vi "MoD Main-Optimize - HPLC ketene2.vi"() -> ()   [LabVIEW 2015]
uses:
  <vilib>/silver_ctls/ArrayMatrixCluster/Real Matrix NI_Silver.ctl
  <vilib>/ni845x/ni845x.llb/ni845xControl.ctl
  <vilib>/MakerHub/LINX/Public/Peripherals/Analog/Analog Read 1 Chan.vi
  <vilib>/MakerHub/LINX/Public/Peripherals/Analog/Analog Read N Chans.vi
  <vilib>/MakerHub/LINX/Public/Peripherals/Digital/Digital Write 1 Chan.vi
  <vilib>/MakerHub/LINX/Private/Local IO/LinxAnalogRead.vi
  <vilib>/MakerHub/LINX/Public/Utilities/Check Channel.vi
  <vilib>/MakerHub/LINX/Public/Peripherals/Digital/Digital Write N Chans.vi
  <vilib>/MakerHub/LINX/Private/Local IO/LinxDigitalWrite.vi
  <vilib>/addons/control/pid/pid.llb/PID Control Input Filter (DBL).vi
  <vilib>/MakerHub/LINX/Private/Utilties/Generate Error.vi
  <vilib>/addons/control/pid/autopid.llb/PID Online Autotuning (Relay Feedback).vi
  <vilib>/Analysis/Matrix/Numeric/Conversions/Array To Matrix - RA2.vi
  <vilib>/ni845x/ni845x.llb/NI-845x Close Device Reference.vi
  <vilib>/addons/control/pid/NI_PID_autopid.lvlib
  <vilib>/addons/control/pid/NI_PID_pid.lvlib
  <vilib>/Analysis/Matrix/NI_Matrix.lvlib
  <vilib>/MakerHub/LINX/LMH-LINX.lvlib
  <instrlib>/Harvard Apparatus PHD Ultra Series/Harvard Apparatus PHD Ultra Series.lvlib
panel:
  out "Temp SS? 6":bool=TRUE
  out "running?":bool=TRUE
  out "new_reactor_volume":bool[](array[boolean])
  out "new_reactor_length":bool[](array[boolean])
  out "Phase_Sensor_voltage":dbl
  out "P_tot":dbl
  out "pause for ms":bool=TRUE
  out "stop_xl_write":bool=TRUE
  out "Num_exp_till_pause":i32
  out "Syringe_pump?":bool=TRUE
  out "System Error":bool=TRUE
  out "error out":errorcluster
  out "Pump setpoint(ul/min) 6":dbl format="%#_13g"
  out "Pump setpoint(ul/min) 5":dbl format="%#_13g"
  out "Pump setpoint(ul/min) 4":dbl format="%#_13g"
  out "Pump setpoint(ul/min) 3":dbl format="%#_13g"
  out "Pump setpoint(ul/min) 2":dbl format="%#_13g"
  out "Pump setpoint(ul/min) 1":dbl format="%#_13g"
  out "Volume (ul) 5":dbl format="%#_13g"
  out "Volume (ul) 4":dbl format="%#_13g"
  out "Volume (ul) 3":dbl format="%#_13g"
  out "Volume (ul) 2":dbl format="%#_13g"
  out "Volume (ul) 1":dbl format="%#_13g"
  in  "tau 5":dbl format="%#_13g"
  out "tau 4":dbl format="%#_13g"
  out "tau 3":dbl format="%#_13g"
  out "tau 2":dbl format="%#_13g"
  out "tau 1":dbl format="%#_13g"
  out "Reactor Length":dbl format="%#_13g"
  out "Flowrate Sensor 2":dbl format="%#_13g"
  out "Flowrate Sensor 1":dbl format="%#_13g"
  out "Pressure 2":dbl format="%#_13g"
  out "Pressure 1":dbl format="%#_13g"
  out "Temperature Control 5":bool=TRUE
  out "Temperature Control 4":bool=TRUE
  out "Temperature Control 3":bool=TRUE
  out "Temperature Control 2":bool=TRUE
  out "Temperature Control 1":bool=TRUE
  out "Temperature SP 5":dbl format="%#_g'C"
  out "Temperature SP 4":dbl format="%#_g'C"
  out "Temperature SP 3":dbl format="%#_g'C"
  out "Temperature SP 2":dbl format="%#_g'C"
  out "Temperature SP 1":dbl format="%#_g'C"
  in  "Bay Temperature 5":dbl
  in  "SSR Duration 5":dbl
  in  "SSR Duration 4":dbl
  in  "SSR Duration 3":dbl
  in  "SSR Duration 2":dbl
  in  "SSR Duration 1":dbl
  in  "Total Product Amount":dbl=1.0 format="%#_gml"
  out "Setup Error":bool=TRUE
  out "Error Message":string
  out "ID CTR":i32
  in  "Tab Control":T1(tab)
  out "Reagent pic 5":picture
  in  "reagent name 5":string="HCl"
  out "Reagent Pic 4":picture
  in  "reagent name 4":string="ethylaluminum dichloride"
  out "Reagent Pic 3":picture
  in  "reagent  name 3":string="cyclohexene"
  in  "Product name":string="55662-89-0"
  in  "reagent name 1":string="Acyl Chloride "
  out "Reagent Pic 1":picture
  in  "Vr5":dbl format="%#_guL"
  in  "Vr4":dbl=400.0 format="%#_guL"
  in  "Vr3":dbl=800.0 format="%#_guL"
  in  "Vr2":dbl format="%#_guL"
  in  "Vr1":dbl format="%#_guL"
  in  "System decide help Button":bool
  in  "Reaction Scheme Confirm":bool
  in  "Synthesis Route Array":string[][](array[string])=[["Acyl Chloride + INTSD", ".5", "PhB(OH)2", "", "", ""], ["Tributyl amine", "4.2", "-", "-", "-", "-"], ["ethylaluminum dichloride", "1", "-", "-", "-", "-"], ["HCl", "", "-", "-", "-", "-"], ["", "", "-", "-", "-", "-"], ["", "", "-", "-", "-", "-"]]
  in  "System decide help Button 2":bool
  out "Setup Confirm":bool=TRUE
  in  "BAY 1":u16(ring) items=["               Bypass", "         Heated Reactor", "    Small Heated Reator", "         Cooled Reactor", "      Packed Bed Reactor", "          Photo Reactor", "             Separator"]
  in  "BAY 5":u16(ring)=6 items=["               Bypass", "         Heated Reactor", "    Small Heated Reactor", "         Cooled Reactor", "     Packed Bed Reactor", "         Photo Reactor", "             Separator"]
  in  "BAY 4":u16(ring)=1 items=["                Bypass", "         Heated Reactor", "    Small Heated Reactor", "         Cooled Reactor", "     Packed Bed Reactor", "         Photo Reactor", "             Separator"]
  in  "BAY 3":u16(ring)=2 items=["               Bypass", "         Heated Reactor", "    Small Heated Reactor", "         Cooled Reactor", "     Packed Bed Reactor", "          Photo Reactor", "             Separator"]
  in  "BAY 2":u16(ring)=2 items=["               Bypass", "         Heated Reactor", "    Small Heated Reactor", "         Cooled Reactor", "      Packed Bed Reactor", "          Photo Reactor", "             Separator"]
  out "Reagent Pic 2":picture
  out "Product Pic":picture
  in  "reagent name 2":string="Tributyl amine"
  in  "reagent name 6":string
  out "Reagent Pic 6":picture
  in  "System Parameters Help Button":bool
  out "Setup Confirm 2":bool
  in  "System Parameters Confirm Button":bool
  in  "Bay Parameters":T2={"Bay 1 "={"Pump 1 Flowrate"=0.0, "optimize_temp"=FALSE, "optimize_tau"=TRUE, "Run at set flowrate"=FALSE, "Pump 2 Flowrate"=0.0, "Temperature Params"=[40.0, 100.0, 100.0], "pump params 1"=[46.3, 463.0, 325.0], "pump params 2"=[11.5, 115.0, 325.0], "Temperature"=0.0, "Run at set temperature"=FALSE}, "Bay 2 "={"Pump 3 Flowrate"=0.0, "optimize_temp"=FALSE, "optimize_tau"=TRUE, "Run at set flowrate"=FALSE, "Temperature Params"=[40.0, 100.0, 100.0], "Resisdence time params"=[4.69, 46.9, 650.0], "pump_at_ratio"=FALSE, "pump_num_ratio"=4.0, "Temperature"=0.0, "Run at set temperature"=FALSE}, "Bay 3 "={"Pump 4 Flowrate"=100.0, "optimize_temp"=TRUE, "optimize_tau"=TRUE, "Run at set flowrate"=FALSE, "Temperature Params"=[30.0, 120.0, 100.0], "Resisdence time params"=[23.15, 231.5, 0.0], "pump_at_ratio"=FALSE, "pump_num_ratio"=1.0, "Temperature "=0.0, "Run at set temperature"=FALSE}, "Bay 4 "={"Pump 5 Flowrate"=40.0, "Run at set flowrate"=FALSE, "optimize_temp"=FALSE, "optimize_tau"=FALSE, "Resisdence time params"=[40.6, 406.0, 225.0], "Temperature Params"=[40.0, 100.0, 80.0], "pump_at_ratio"=FALSE, "pump_num_ratio"=2.0, "Temperature"=0.0, "Run at set temperature"=FALSE}, "Bay 5 "={"Pump 6 Flowrate"=0.0, "Run at set flowrate"=FALSE, "optimize_temp"=FALSE, "optimize_tau"=FALSE, "Resisdence time params"=[7.62, 114.27, 0.0], "Temperature Params"=[0.0, 0.0, 0.0], "pump_at_ratio"=TRUE, "pump_num_ratio"=2.0, "Temperature"=0.0, "Run at set temperature"=FALSE}, "Excel File Name"="C:\\Users\\HPLC\\Dropbox (MIT)\\MoD Files\\Data\\Ketene04222018", "hplc File Name"="C:\\Chem32\\1\\Data\\MOD", "Matlab File"="C:\\Users\\HPLC\\Dropbox (MIT)\\MoD Files\\Data\\Ketene04222018_1", "Syringe for Pump 2?"=TRUE, "Num_conditons_per_wait"=2.0, "Continue from previous optimization?"=FALSE, "Total Number of Experiments 2"=45.0, "Hplc Wait time(min)"=14.0, "increas_decrease_hplc_peak"=FALSE, "Internal Standard?"=TRUE, "ISTD start"=5.0, "ISTD end"=6.0, "hplc_start"=13.0, "hplc_end"=13.45, "throughput_yield"=TRUE} {"Hplc Wait time(min)" format="%#_13g"; "Bay 5"."Temperature Params" format="%#_g'C"; "Bay 4"."Temperature Params" format="%#_g'C"; "Bay 3"."Temperature Params" format="%#_g'C"; "Bay 2"."Temperature Params" format="%#_g'C"; "Bay 1"."Temperature Params" format="%#_g'C"}
  out "System Confirm Not Clicked":string
  out "best_exp_num":dbl=1.0
  out "temperature_best":dbl[](array[numeric])
  out "Flowrates(ul/min)_best":dbl[](array[numeric])
  out "System Status":u16(ring)=2 caption="Sy" items=["System  Error", "System Running", "System Standby"]
  out "Current Experiment":dbl=1.0
  out "Total Number of Experiments":dbl=33.0
  out "Phase Sensor Chart":T3(graph)
  out "HPLC Analysis":bool
  out "Equlibrating Temperature":bool
  out "Flushing System":bool
  out "Calculate condition":bool
  out "Temperature 5":dbl format="%#_g'C"
  out "Temperature 4":dbl format="%#_g'C"
  out "Temperature 3":dbl format="%#_g'C"
  out "Temperature 2":dbl format="%#_g'C"
  out "Temperature 1":dbl format="%#_g'C"
  out "Flowrate Chart":T4(graph)
  out "Teperature Chart":T3(graph)
  out "Pump Setpoints Chart":T3(graph)
  out "Pressure Chart":T3(graph)
  out "Optimization_loop_index":i32
  out "curr_wait_time":dbl
  out "total_flush_time":dbl
  out "Temp SS? 5":bool=TRUE
  out "Temp SS? 4":bool=TRUE
  out "Temp SS? 3":bool=TRUE
  out "Temp SS? 2":bool=TRUE
  out "Temp SS? 1":bool=TRUE
  out "System Flushed?":bool
  out "stop_button clicked":bool
  in  "Pump Addresses":string[](array[string])=["g", "e", "j", "i", "f", "h"]
  out "experiment history":T5
  in  "Number of System Flushes per condtion":dbl=2.5
  in  "calculate volume 3":bool=TRUE
  in  "calculate volume 2":bool=TRUE
  in  "calculate volume 1":bool=TRUE
  in  "calculate volume 4":bool=TRUE
  in  "calculate volume 5":bool
  in  "Extra system dead volume":dbl format="%#_gul"
  in  "new reactor length? 1":bool
  in  "tube_length(in)":dbl[](array[numeric])=[188.0, 188.0, 10.0, 10.0, 10.0]
  out "Pause Before Analysis":bool
  out "Chiller COMM Port":bool
  out "Arduino COMM Port 2":bool
  out "Temperature Sensor COMM Port":bool
  out "Flow Rate":bool
  out "Pressure":bool
  out "Pump COMM Port":bool
  in  "COMM Port :: Milligat Pumps":refnum<visa-resource-name>="COM10"
  in  "Arduino COMM Port":refnum<visa-resource-name>="COM3"
  in  "Sample Valve COMM::Port":refnum<visa-resource-name>="COM4"
  in  "COMM Port:: Harvard Syringe Pump":refnum<visa-resource-name>="COM5"
  in  "tube_id(in)":enum16{".01", ".02", ".03", ".04"}[](array[ring])=[enum.".03", enum.".03", enum.".03", enum.".03", enum.".03"]
  out "Total System Resisdence Time(min)":dbl
  in  "Debug_run_button":bool
  in  "new reactor length? 2":bool
  in  "new reactor length? 3":bool
  in  "new reactor length? 4":bool
  in  "new reactor length? 5":bool
  in  "IR Sensor Device":T6="USB0::0x3923::0x7514::01B3FF21::RAW"
  out "Stop":bool=TRUE
  in  "Run_Stop_cluster":T7
  # "Molecules on Demand"
  # "Synthetic Route"
  # "5"
  # "6"
  # "4"
  # "Product"
  # "1"
  # "2"
  # "3"
  # "Reagent List"
  # "Concentration(M)"
  # "Molecule"
  # "1"
  # "1"
  # "2"
  # "2"
  # "3"
  # "3"
  # "4"
  # "4"
  # "5"
  # "6"
  # "5"
  # "6"
  # "Product"
  # "Reactor Volume:"
  # "Optimization Parameters"
  # "Pause after"
  # "Experiments"
  # "Optimize for"
  # "to"
  # "of HPLC Peak from"
  # "from"
  # "to"
  # "min"
  # "min"
  # "HPLC runtime"
  # "# Iterations"
  # "Reporting"
  # "Excel Output File Name"
  # "HPLC File Path"
  # "MATLAB File Path"
  # "Temperature"
  # "Flowrate(ul/min)"
  # "Lower Bound"
  # "Upper Bound"
  # "Optimize?"
  # "-or-"
  # "Run at"
  # "times incoming flow"
  # "Setpoint"
  # "Temperature"
  # "Flowrate(ul/min)"
  # "Lower Bound"
  # "Upper Bound"
  # "Optimize?"
  # "-or-"
  # "Run at"
  # "times incoming flow"
  # "Setpoint"
  # "Temperature"
  # "Flowrate(ul/min)"
  # "Lower Bound"
  # "Upper Bound"
  # "Optimize?"
  # "-or-"
  # "Run at"
  # "times incoming flow"
  # "Setpoint"
  # "Temperature"
  # "Flowrate 3 (ul/min)"
  # "Lower Bound"
  # "Upper Bound"
  # "Optimize?"
  # "-or-"
  # "Run at"
  # "times incoming flow"
  # "Setpoint"
  # "Temperature"
  # "Flowrate 1(ul/min)"
  # "Flowrate 2(ul/min)"
  # "Lower Bound"
  # "Upper Bound"
  # "Optimize?"
  # "Setpoint"
  # "Pressure (psi)"
  # "System Status"
  # "Temperature('C)"
  # "BAY"
  # "1"
  # "2"
  # "3"
  # "4"
  # "5"
  # "Pump Flowrate Setpoint(ul/min)"
  # "Flowrate (ul/min)"
  # "Phase Sensor"
  # "Current Experiment"
  # "Temperature('C)"
  # "Flowrate(ul/min)"
  # "Exp"
  # "Current Best Condition"
  # "Time to reach steady state:"
  # "Current Wait Time:"
  # "Experimental Steps"
  # "Calculated New Conditions"
  # "Steady State"
  # "Analyzed HPLC"
  # "Equilibrated Temperature"
  # "Tube Length (cm)"
  # "Bay"
  # "Tube ID (in)"
  # "Calculate Volume"
  # "Use new tube length"
  # "1."
  # "2."
  # "3."
  # "4."
  # "5."
  # "Reactor Lengths\n*Heated Reactor - 188cm * Small Reactor - 99cm * Bypass - 10cm * Separator - *"
  # "1"
  # "2"
  # "3"
  # "4"
  # "5"
  # "All Experimental Data"
  # "6"
  # "P1"
  # "P2"
  # "P3"
  # "P4"
  # "P5"
  # "P6"
  # "T1"
  # "T2"
  # "T3"
  # "T4"
  # "T5"
  # "Obj_fun"
  # "HPLC_Data"
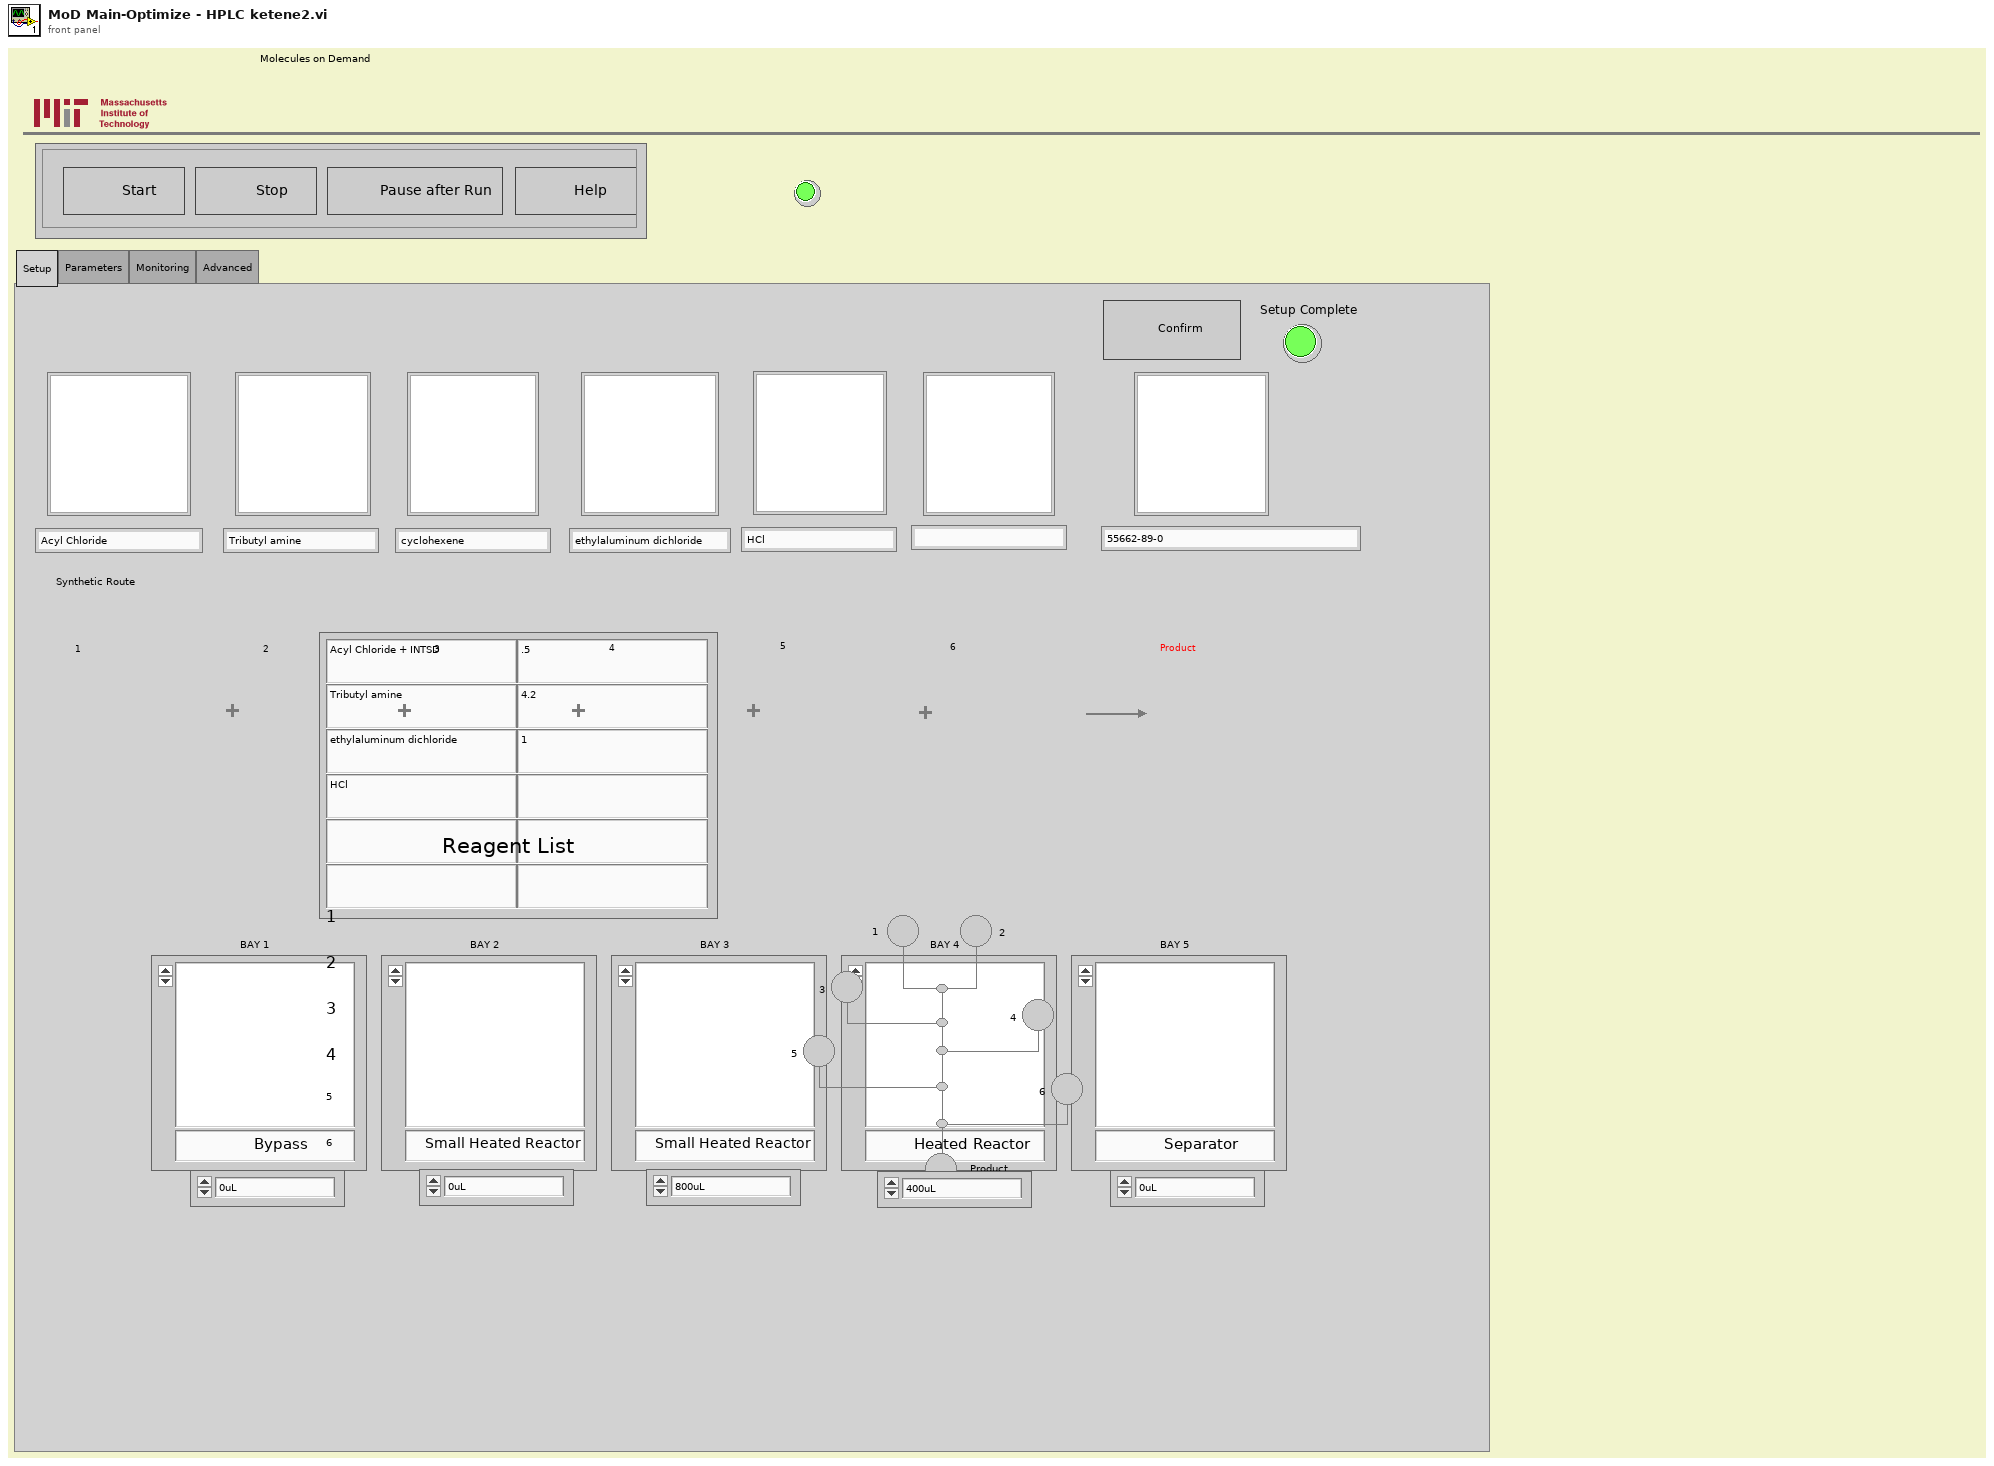
[diagram p1: front panel]
types:
  T1 = enum32{"Setup", "Parameters", "Monitoring", "Advanced"}
  T2 = cluster{"Bay 1 ":cluster{"Pump 1 Flowrate":dbl, "optimize_temp":bool, "optimize_tau":bool, "Run at set flowrate":bool, "Pump 2 Flowrate":dbl, "Temperature Params":dbl[], "pump params 1":dbl[], "pump params 2":dbl[], "Temperature":dbl, "Run at set temperature":bool}, "Bay 2 ":cluster{"Pump 3 Flowrate":dbl, "optimize_temp":bool, "optimize_tau":bool, "Run at set flowrate":bool, "Temperature Params":dbl[], "Resisdence time params":dbl[], "pump_at_ratio":bool, "pump_num_ratio":dbl, "Temperature":dbl, "Run at set temperature":bool}, "Bay 3 ":cluster{"Pump 4 Flowrate":dbl, "optimize_temp":bool, "optimize_tau":bool, "Run at set flowrate":bool, "Temperature Params":dbl[], "Resisdence time params":dbl[], "pump_at_ratio":bool, "pump_num_ratio":dbl, "Temperature ":dbl, "Run at set temperature":bool}, "Bay 4 ":cluster{"Pump 5 Flowrate":dbl, "Run at set flowrate":bool, "optimize_temp":bool, "optimize_tau":bool, "Resisdence time params":dbl[], "Temperature Params":dbl[], "pump_at_ratio":bool, "pump_num_ratio":dbl, "Temperature":dbl, "Run at set temperature":bool}, "Bay 5 ":cluster{"Pump 6 Flowrate":dbl, "Run at set flowrate":bool, "optimize_temp":bool, "optimize_tau":bool, "Resisdence time params":dbl[], "Temperature Params":dbl[], "pump_at_ratio":bool, "pump_num_ratio":dbl, "Temperature":dbl, "Run at set temperature":bool}, "Excel File Name":string, "hplc File Name":string, "Matlab File":string, "Syringe for Pump 2?":bool, "Num_conditons_per_wait":dbl, "Continue from previous optimization?":bool, "Total Number of Experiments 2":dbl, "Hplc Wait time(min)":dbl, "increas_decrease_hplc_peak":bool, "Internal Standard?":bool, "ISTD start":dbl, "ISTD end":dbl, "hplc_start":dbl, "hplc_end":dbl, "throughput_yield":bool}
  T3 = cluster{"[0]":dbl, "[1]":dbl, "[2]":dbl, "[3]":dbl, "[4]":dbl, "[5]":dbl, "[6]":dbl, "[7]":dbl, "[8]":dbl}
  T4 = cluster{"[0]":i32, "[1]":i32, "[2]":i32, "[3]":i32, "[4]":i32, "[5]":i32, "[6]":i32, "[7]":i32, "[8]":i32}
  T5 = typedef "Real Matrix NI_Silver.ctl" = dbl[][]
  T6 = typedef "ni845xControl.ctl" = refnum<k21>
  T7 = cluster{"Stop":bool, "Run":bool, "Stop Run Button":bool, "Help Button":bool}
  T8 = cluster{"Proportional gain Kc":dbl, "Integral time Ti (sec)":dbl, "Derivative time Ti (sec)":dbl}
  T9 = cluster{"type of controller":enum16{"P", "PI", "PID"}, "relay cycles":i32, "relay amplitude":dbl, "control specifications":enum16{"Fast", "Normal", "Slow"}, "PV noise level":dbl}
  T10 = typedef "LMH-LINX.lvlib/LINX Ref.ctl" = cluster{"IO":T11, "Interface":T12, "LINX Device Config":T13}
  T11 = typedef "LMH-LINX.lvlib/Platform.ctl" = enum16{"Remote", "Local"}
  T12 = typedef "LMH-LINX.lvlib/Interface.ctl" = enum16{"Serial", "TCP"}
  T13 = typedef "LMH-LINX.lvlib/Device.lvlib/LINX Device Config.ctl" = cluster{"Interface":T12, "COM Port":refnum<visa-resource-name>, "TCP Configuration":T14, "Device Family":u8, "Device ID":u8, "Device Name":string, "TCP Ref":refnum<k5>, "Channels":T15}
  T14 = typedef "LMH-LINX.lvlib/Device.lvlib/TCP Config.ctl" = cluster{"IP Address":string, "Port":u16}
  T15 = typedef "LMH-LINX.lvlib/Channels.ctl" = cluster{"DI":u8[], "DO":u8[], "AI":u8[], "AO":u8[], "PWM":u8[], "QE":u8[], "UART":u8[], "I2C 2":u8[], "SPI":u8[], "CAN":u8[], "Servo":u8[], "AI Ref (V)":dbl, "AI Resolution (Bits)":u8, "AO Ref (V)":dbl, "AO Resolution (Bits)":u8}
  T16 = typedef "imagedata.ctl" = cluster{"image type":i32, "image depth":i32, "image":u8[], "mask":u8[], "colors":u32[], "Rectangle":cluster{"left":i16, "top":i16, "right":i16, "bottom":i16}}
  T17 = cluster{"proportional gain (Kc)":dbl, "integral time (Ti, min)":dbl, "derivative time (Td, min)":dbl}
  T18 = typedef "NI_Matrix.lvlib/RealMatrix.ctl" = dbl[][]
  T19 = enum16{"Left Button", "Center Button", "Right Button", "Window Close"}
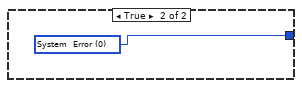
[diagram p4: hidden frame]
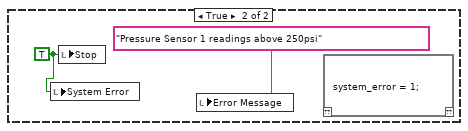
[diagram p6: hidden frame]
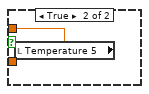
[diagram p7: hidden frame]
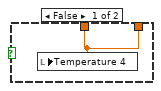
[diagram p8: hidden frame]
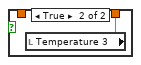
[diagram p9: hidden frame]
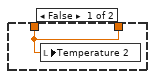
[diagram p10: hidden frame]
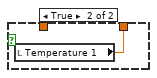
[diagram p11: hidden frame]
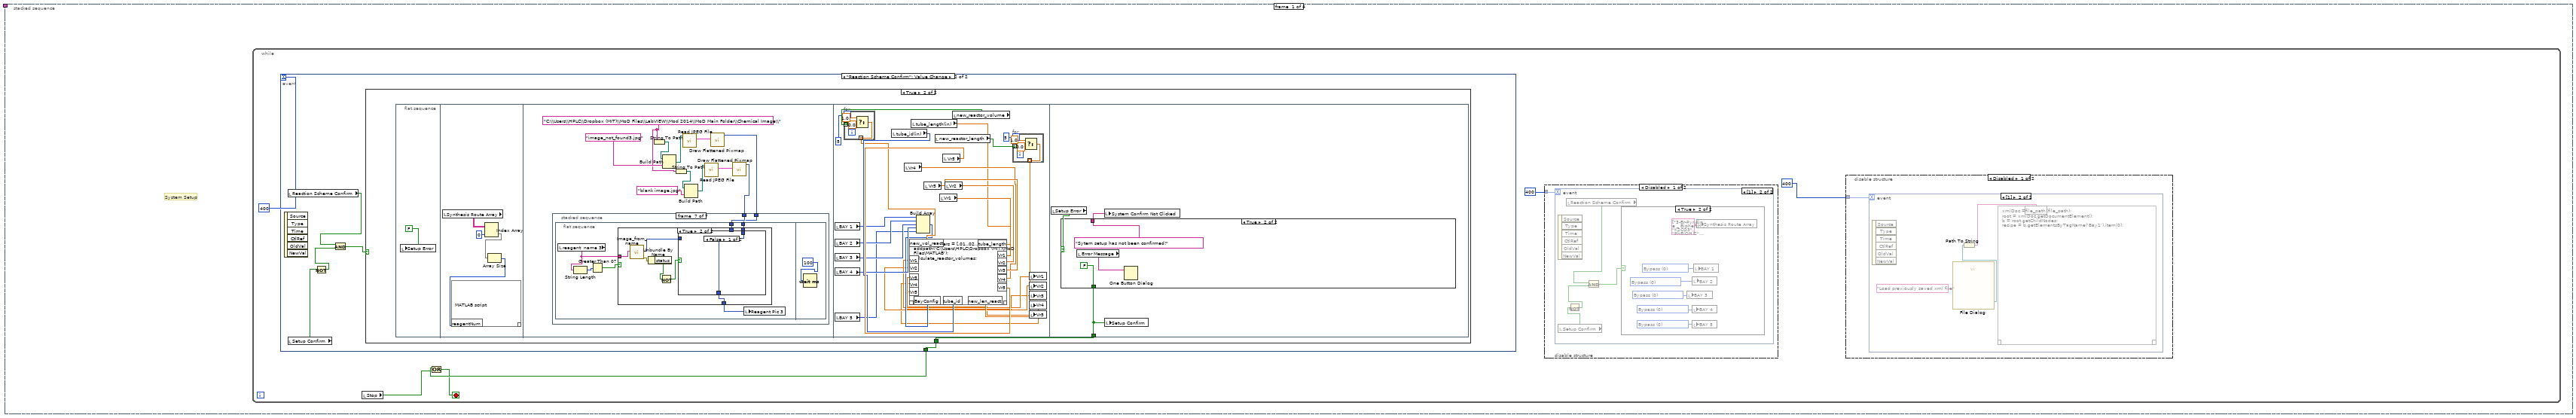
[diagram p12: hidden frame]
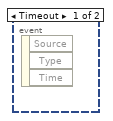
[diagram p13: hidden frame]
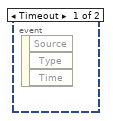
[diagram p15: hidden frame]
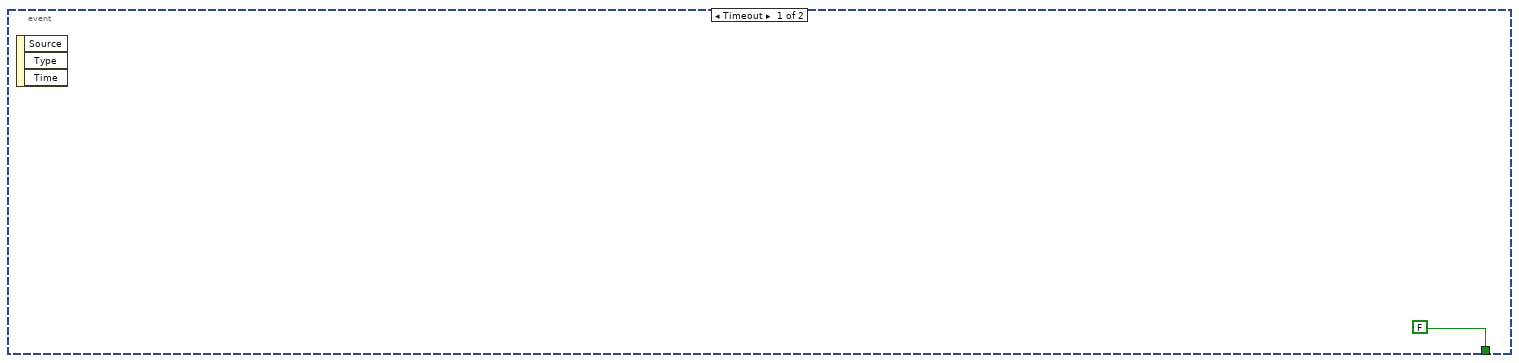
[diagram p18: hidden frame]
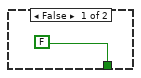
[diagram p19: hidden frame]
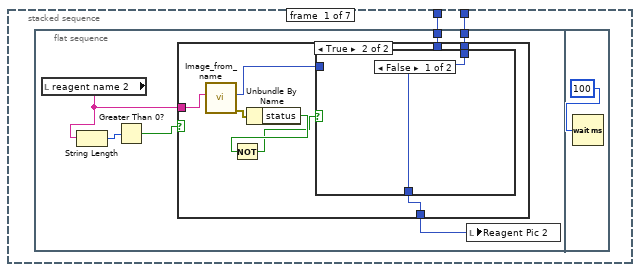
[diagram p20: hidden frame]
diagram:
  # "Assume User always uses the first bay first"
  n1 = flat-sequence {
    tunnel: ["COMM Port :: Milligat Pumps"] -> w9
    tunnel: ["Arduino COMM Port"] -> w8
    tunnel: [w11] -> w5
    tunnel: ["Bay Parameters"] -> w4
    tunnel: [w60] -> w10
    tunnel: w9 -> [w60]
    tunnel: w8 -> [w48]
    tunnel: [w54] -> w7
    tunnel: [w52] -> w6
    tunnel: w5 -> [w52]
    tunnel: w4 -> [w50]
    tunnel: [w47] -> w3
    tunnel: w10 -> [w66]
    tunnel: w7 -> [w65]
    tunnel: w6 -> [w63]
    tunnel: w3 -> [w61]
    tunnel: [w61] -> w1
    tunnel: [w1409] -> w2
    tunnel: w1 -> [w1409]
    tunnel: w2 -> [w1410]
    frame #0 {
      w36 = FALSE ("Equlibrating Temperature")
      n2 = script code="TempArr1=[23 23 23 23 23 23 23 23 23 23]';\nTempArr2=[23 23 23 23 23 23 23 23 23 23]';\nTempArr3=[23 23 23 23 23 23 23 23 23 23]';\nTempArr4=[23 23 23 23 23 23 23 23 23 23]';\nTempArr5=[23 23 23 23 23 23 23 23 23 23]';\nTempArrLED=[23 23 23 23 23 23 23 23 23 23]';\ntemp_error1 =0;\ntemp_error2 =0;\ntemp_error3 =0;\ntemp_error4 =0;\ntemp_error5 =0;\ntemp_check1 = 0;\ntemp_check2 = 0;\ntemp_check3 = 0;\ntemp_check4 = 0;\ntemp_check5 = 0;\nT1=23;\nT2=23;\nT3=23;\nT4=23;\nT5=23;"() -> ()  [unwired: 1 in, 1 out]
      n3 = Build Array("calculate volume 1", "calculate volume 2", "calculate volume 3", "calculate volume 4", "calculate volume 5") -> (→"new_reactor_volume":bool[])
      n4 = Build Array("new reactor length? 1", "new reactor length? 2", "new reactor length? 3", "new reactor length? 4", "new reactor length? 5") -> (→"new_reactor_length":bool[])
      n5 = call <vilib>:"Initialize.vi"("VISA resource name"="COMM Port:: Harvard Syringe Pump") -> ("VISA resource name out"=w11:refnum<visa-resource-name>)  [unwired: 9 in, 1 out]
      "Stop" <- FALSE ("Stop")
      "ID CTR" <- 0
      "Setup Confirm" <- FALSE ("Setup Confirm")
      "Error Message" <- "System shutdown sucessfully. No errors to report." ("Error Message")
      "Setup Error" <- FALSE ("Setup Error")
      "Reactor Length" <- 10.5
      "System Error" <- FALSE ("System Error")
      "Num_exp_till_pause" <- 0 ("Num_exp_till_pause")
      "Equlibrating Temperature" <- w36
      "Calculate condition" <- w36
      "Flushing System" <- w36
      "HPLC Analysis" <- w36
      "stop_xl_write" <- FALSE ("stop_xl_write")
      "Pump setpoint(ul/min) 1" <- 0.0 ("Pump setpoint(ul/min) 1")
      "Pump setpoint(ul/min) 2" <- 0.0 ("Pump setpoint(ul/min) 2")
      "Pump setpoint(ul/min) 4" <- 0.0 ("Pump setpoint(ul/min) 4")
      "Pump setpoint(ul/min) 6" <- 0.0 ("Pump setpoint(ul/min) 6")
      "Pump setpoint(ul/min) 3" <- 0.0 ("Pump setpoint(ul/min) 3")
      "Pump setpoint(ul/min) 5" <- 0.0 ("Pump setpoint(ul/min) 5")
      "pause for ms" <- FALSE ("pause for ms")
      "Setup Confirm 2" <- FALSE ("Setup Confirm 2")
      "running?" <- FALSE ("running?")
    }
    frame #1 {
      w49 = FALSE
      w59 = 23
      (unwired) path "C:/Users/User1/Documents/Lab/MoD/Images"
      n6 = disable-structure shown="Disabled" {
        frame Disabled {
          n7 = local read "BAY 2"() -> ()  [unwired: 1 out]
          n8 = local read "BAY 3"() -> ()  [unwired: 1 out]
          n9 = local read "BAY 4"() -> ()  [unwired: 1 out]
          n10 = local read "BAY 5"() -> ()  [unwired: 1 out]
          n11 = local read "BAY 1"() -> ()  [unwired: 1 out]
        }
        frame Enabled {
        }
      }
      n12 = local write "Debug_run_button"(TRUE) -> ()
      n13 = call <vilib>:"Initialize.vi"("Serial Port"=w48) -> ("LINX Resource"=w47:T10)  [unwired: 8 in, 2 out]
      n14 = local write "System Parameters Confirm Button"(w49) -> ()
      n15 = local write "Setup Confirm 2"(w49) -> ()
      n16 = Unbundle By Name(w50) -> ("Syringe for Pump 2?"=→"Syringe_pump?":bool)
      n17 = local write "Temperature 1"(w59) -> ()
      n18 = local write "Temperature 2"(w59) -> ()
      n19 = local write "Temperature 3"(w59) -> ()
      n20 = local write "Temperature 4"(w59) -> ()
      n21 = local write "Temperature 5"(w59) -> ()
      n22 = local write "Temperature SP 1"(w59) -> ()
      n23 = local write "Temperature SP 2"(w59) -> ()
      n24 = local write "Temperature SP 3"(w59) -> ()
      n25 = local write "Temperature SP 4"(w59) -> ()
      n26 = local write "Temperature SP 5"(w59) -> ()
      n27 = Current VI's Path() -> (path=w58:path)
      n28 = Strip Path(path=w58) -> (stripped path=w56:path)  [unwired: 1 out]
      n29 = Strip Path(path=w56) -> (stripped path=w55:path)  [unwired: 1 out]
      n30 = Build Path(base path=w55, name or relative path="MATLAB") -> (appended path=w54:path)
    }
    frame #2 {
      # "Main Help Dialog Popup"
      n31 = while {
        stop <- w1403 stop-if-true
        n32 = event shown="[6] \"Run_Stop_cluster.Run\": Value Change" {
          selector: _ -> [_ _ _ _ _ _ _]
          dyn-events: _ -> [_ _ _ _ _ _ _]
          timeout: 100 -> [_ _ _ _ _ _ _]
          event Timeout {
            n33 = event-data() -> ()  [unwired: 1 in, 3 out]
          }
          event "Run_Stop_cluster.Help Button": Value Change {
            n34 = local read "Run_Stop_cluster"() -> (w1406:T7)
            n35 = event-data() -> ()  [unwired: 1 in, 4 out]
            n36 = Unbundle By Name(w1406) -> ("Help Button"=w1405:bool)
            n37 = case shown="True" w1405 {
              frame False {
              }
              frame True {
                n38 = call "help.vi"() -> ()  [unwired: 11 in]
              }
            }
          }
          event "System decide help Button": Value Change {
            n39 = event-data() -> ()  [unwired: 1 in, 5 out]
            n40 = call "help_synthesis_man-auto_instructions.vi"() -> ()  [unwired: 12 in]
          }
          event "System Parameters Help Button": Value Change {
            n41 = event-data() -> ()  [unwired: 1 in, 5 out]
            n42 = call "help_parameters_setup.vi"() -> ()  [unwired: 12 in]
          }
          event "System decide help Button 2": Value Change {
            n43 = event-data() -> ()  [unwired: 1 in, 5 out]
            n44 = call "help_synthesis_route_instructions.vi"() -> ()  [unwired: 12 in]
          }
          event "Run_Stop_cluster.Stop": Value Change {
            n45 = event-data() -> ()  [unwired: 1 in, 5 out]
            n46 = local write "Stop"(TRUE) -> ()
          }
          event "Run_Stop_cluster.Run": Value Change {
            n47 = event-data() -> ()  [unwired: 1 in, 5 out]
            n48 = local write "running?"(TRUE) -> ()
          }
        }
        n49 = local read "Stop"() -> (w1403:bool)
      }
      n50 = stacked-sequence {
        tunnel: w66 -> [_ _ _ _]
        tunnel: w65 -> [_ w432 _ _]
        tunnel: w63 -> [_ _ _ w599]
        tunnel: w61 -> [_ _ _ w597]
        frame #0 {
          # "System Setup"
          n51 = while {
            stop <- w207 stop-if-true
            n52 = event shown="[1] \"Reaction Scheme Confirm\": Value Change" {
              selector: _ -> [_ _]
              dyn-events: _ -> [_ _]
              timeout: 400 -> [_ _]
              tunnel: [FALSE w227] -> w209
              event Timeout {
                n53 = event-data() -> ()  [unwired: 1 in, 3 out]
              }
              event "Reaction Scheme Confirm": Value Change {
                n54 = event-data() -> ()  [unwired: 1 in, 6 out]
                n55 = local read "Reaction Scheme Confirm"() -> (w231:bool)
                n56 = local read "Setup Confirm"() -> (w229:bool)
                n57 = Not(x=w229) -> (.not. x?=w228:bool)
                n58 = And(x=w231, y=w228) -> (x .and. y?=w230:bool)
                n59 = case shown="True" w230 {
                  tunnel: [FALSE w233] -> w227
                  frame False {
                  }
                  frame True {
                    n60 = flat-sequence {
                      tunnel: [w422] -> w233
                      frame #0 {
                        n61 = local write "Setup Error"(FALSE) -> ()
                      }
                      frame #1 {
                        n62 = local read "Synthesis Route Array"() -> (w237:string[][])
                        n63 = Index Array(array=w237, index (col)=0 ("disabled index (col)")) -> (element=w235:string[])  [unwired: 1 in]
                        n64 = Array Size(array=w235) -> (size(s)=w238:i32)
                        n65 = script code="MATLAB script"("reagentNum"=w238) -> ()  [unwired: 1 in, 1 out]
                      }
                      frame #2 {
                        w241 = "C:\\Users\\HPLC\\Dropbox (MIT)\\MoD Files\\LabVIEW\\Mod 2014\\MoD Main Folder\\Chemical Image\\" ("string")
                        n66 = String To Path(string=w241) -> (path=w247:path)
                        n67 = Build Path(base path=w247, name or relative path="image_not_found3.jpg") -> (appended path=w246:path)
                        n68 = String To Path(string=w241) -> (path=w244:path)
                        n69 = call <vilib>:"Read JPEG File.vi"("path to JPEG file"=w246) -> ("image data"=w249:T16)  [unwired: 1 in, 9 out]
                        n70 = Build Path(base path=w244, name or relative path="blank image.jpg") -> (appended path=w242:path)
                        n71 = call <vilib>:"Read JPEG File.vi"("path to JPEG file"=w242) -> ("image data"=w245:T16)  [unwired: 1 in, 9 out]
                        n72 = call <vilib>:"Draw Flattened Pixmap.vi"("image data"=w249) -> ("new picture"=w240:picture)  [unwired: 3 in, 5 out]
                        n73 = call <vilib>:"Draw Flattened Pixmap.vi"("image data"=w245) -> ("new picture"=w239:picture)  [unwired: 3 in, 5 out]
                        n74 = stacked-sequence {
                          tunnel: w240 -> [w251 w271 w291 w311 w331 w350 w370]
                          tunnel: w239 -> [w250 w270 w290 w310 w330 w351 w371]
                          frame #0 {
                            n75 = flat-sequence {
                              tunnel: w251 -> [w257]
                              tunnel: w250 -> [w255]
                              frame #0 {
                                n76 = local read "reagent name 2"() -> (w253:string)
                                n77 = String Length(string=w253) -> (length=w256:i32)
                                n78 = Greater Than 0?(x=w256) -> (x > 0?=w254:bool)
                                n79 = case shown="True" w254 {
                                tunnel: w257 -> [_ w263]
                                tunnel: w255 -> [w258 _]
                                tunnel: [w258 w262] -> w252
                                tunnel: w253 -> [_ w261]
                                frame False {
                                }
                                frame True {
                                n80 = call "Image_from_name.vi"("Chemical Name"=w261) -> ("error out"=w264:errorcluster, "Downloaded Picture"=w265:picture)  [unwired: 8 in, 1 out]
                                n81 = Unbundle By Name(w264) -> ("status"=w260:bool)
                                n82 = Not(x=w260) -> (.not. x?=w259:bool)
                                n83 = case shown="False" w259 {
                                tunnel: w265 -> [_ w268]
                                tunnel: [w266 w267] -> w262
                                tunnel: w263 -> [w266 _]
                                frame False {
                                }
                                frame True {
                                n84 = call <vilib>:"Draw Flattened Pixmap.vi"("picture"=w268) -> ("new picture"=w267:picture)  [unwired: 8 in]
                                }
                                }
                                }
                                }
                                n85 = local write "Reagent Pic 2"(w252) -> ()
                              }
                              frame #1 {
                                n86 = Wait (ms)(milliseconds to wait=100) -> ()  [unwired: 1 out]
                              }
                            }
                          }
                          frame #1 {
                            n87 = flat-sequence {
                              tunnel: w271 -> [w277]
                              tunnel: w270 -> [w275]
                              frame #0 {
                                n88 = local read "reagent name 1"() -> (w272:string)
                                n89 = String Length(string=w272) -> (length=w276:i32)
                                n90 = Greater Than 0?(x=w276) -> (x > 0?=w274:bool)
                                n91 = case shown="True" w274 {
                                tunnel: w277 -> [_ w283]
                                tunnel: w275 -> [w278 _]
                                tunnel: [w278 w282] -> w273
                                tunnel: w272 -> [_ w281]
                                frame False {
                                }
                                frame True {
                                n92 = call "Image_from_name.vi"("Chemical Name"=w281) -> ("error out"=w284:errorcluster, "Downloaded Picture"=w285:picture)  [unwired: 8 in, 1 out]
                                n93 = Unbundle By Name(w284) -> ("status"=w280:bool)
                                n94 = Not(x=w280) -> (.not. x?=w279:bool)
                                n95 = case shown="True" w279 {
                                tunnel: w285 -> [_ w288]
                                tunnel: [w286 w287] -> w282
                                tunnel: w283 -> [w286 _]
                                frame False {
                                }
                                frame True {
                                n96 = call <vilib>:"Draw Flattened Pixmap.vi"("picture"=w288) -> ("new picture"=w287:picture)  [unwired: 8 in]
                                }
                                }
                                }
                                }
                                n97 = local write "Reagent Pic 1"(w273) -> ()
                              }
                              frame #1 {
                                n98 = Wait (ms)(milliseconds to wait=100) -> ()  [unwired: 1 out]
                              }
                            }
                          }
                          frame #2 {
                            n99 = flat-sequence {
                              tunnel: w291 -> [w297]
                              tunnel: w290 -> [w295]
                              frame #0 {
                                n100 = local read "Product name"() -> (w292:string)
                                n101 = String Length(string=w292) -> (length=w296:i32)
                                n102 = Greater Than 0?(x=w296) -> (x > 0?=w294:bool)
                                n103 = case shown="True" w294 {
                                tunnel: w297 -> [_ w303]
                                tunnel: w295 -> [w298 _]
                                tunnel: [w298 w302] -> w293
                                tunnel: w292 -> [_ w301]
                                frame False {
                                }
                                frame True {
                                n104 = call "Image_from_name.vi"("Chemical Name"=w301) -> ("error out"=w304:errorcluster, "Downloaded Picture"=w305:picture)  [unwired: 8 in, 1 out]
                                n105 = Unbundle By Name(w304) -> ("status"=w299:bool)
                                n106 = Not(x=w299) -> (.not. x?=w300:bool)
                                n107 = case shown="False" w300 {
                                tunnel: w305 -> [_ w308]
                                tunnel: [w306 w307] -> w302
                                tunnel: w303 -> [w306 _]
                                frame False {
                                }
                                frame True {
                                n108 = call <vilib>:"Draw Flattened Pixmap.vi"("picture"=w308) -> ("new picture"=w307:picture)  [unwired: 8 in]
                                }
                                }
                                }
                                }
                                n109 = local write "Product Pic"(w293) -> ()
                              }
                              frame #1 {
                                n110 = Wait (ms)(milliseconds to wait=100) -> ()  [unwired: 1 out]
                              }
                            }
                          }
                          frame #3 {
                            n111 = flat-sequence {
                              tunnel: w311 -> [w317]
                              tunnel: w310 -> [w315]
                              frame #0 {
                                n112 = local read "reagent name 6"() -> (w312:string)
                                n113 = String Length(string=w312) -> (length=w316:i32)
                                n114 = Greater Than 0?(x=w316) -> (x > 0?=w314:bool)
                                n115 = case shown="True" w314 {
                                tunnel: w317 -> [_ w323]
                                tunnel: w315 -> [w318 _]
                                tunnel: [w318 w322] -> w313
                                tunnel: w312 -> [_ w321]
                                frame False {
                                }
                                frame True {
                                n116 = call "Image_from_name.vi"("Chemical Name"=w321) -> ("error out"=w324:errorcluster, "Downloaded Picture"=w325:picture)  [unwired: 8 in, 1 out]
                                n117 = Unbundle By Name(w324) -> ("status"=w319:bool)
                                n118 = Not(x=w319) -> (.not. x?=w320:bool)
                                n119 = case shown="False" w320 {
                                tunnel: w325 -> [_ w328]
                                tunnel: [w326 w327] -> w322
                                tunnel: w323 -> [w326 _]
                                frame False {
                                }
                                frame True {
                                n120 = call <vilib>:"Draw Flattened Pixmap.vi"("picture"=w328) -> ("new picture"=w327:picture)  [unwired: 8 in]
                                }
                                }
                                }
                                }
                                n121 = local write "Reagent Pic 6"(w313) -> ()
                              }
                              frame #1 {
                                n122 = Wait (ms)(milliseconds to wait=100) -> ()  [unwired: 1 out]
                              }
                            }
                          }
                          frame #4 {
                            n123 = flat-sequence {
                              tunnel: w331 -> [w337]
                              tunnel: w330 -> [w335]
                              frame #0 {
                                n124 = local read "reagent name 5"() -> (w332:string)
                                n125 = String Length(string=w332) -> (length=w336:i32)
                                n126 = Greater Than 0?(x=w336) -> (x > 0?=w334:bool)
                                n127 = case shown="True" w334 {
                                tunnel: w337 -> [_ w343]
                                tunnel: w335 -> [w338 _]
                                tunnel: [w338 w342] -> w333
                                tunnel: w332 -> [_ w341]
                                frame False {
                                }
                                frame True {
                                n128 = call "Image_from_name.vi"("Chemical Name"=w341) -> ("error out"=w344:errorcluster, "Downloaded Picture"=w345:picture)  [unwired: 8 in, 1 out]
                                n129 = Unbundle By Name(w344) -> ("status"=w339:bool)
                                n130 = Not(x=w339) -> (.not. x?=w340:bool)
                                n131 = case shown="False" w340 {
                                tunnel: w345 -> [_ w348]
                                tunnel: [w346 w347] -> w342
                                tunnel: w343 -> [w346 _]
                                frame False {
                                }
                                frame True {
                                n132 = call <vilib>:"Draw Flattened Pixmap.vi"("picture"=w348) -> ("new picture"=w347:picture)  [unwired: 8 in]
                                }
                                }
                                }
                                }
                                n133 = local write "Reagent pic 5"(w333) -> ()
                              }
                              frame #1 {
                                n134 = Wait (ms)(milliseconds to wait=100) -> ()  [unwired: 1 out]
                              }
                            }
                          }
                          frame #5 {
                            n135 = flat-sequence {
                              tunnel: w351 -> [w355]
                              tunnel: w350 -> [w354]
                              frame #0 {
                                n136 = local read "reagent name 4"() -> (w352:string)
                                n137 = String Length(string=w352) -> (length=w357:i32)
                                n138 = Greater Than 0?(x=w357) -> (x > 0?=w356:bool)
                                n139 = case shown="True" w356 {
                                tunnel: w354 -> [_ w363]
                                tunnel: w355 -> [w358 _]
                                tunnel: [w358 w362] -> w353
                                tunnel: w352 -> [_ w361]
                                frame False {
                                }
                                frame True {
                                n140 = call "Image_from_name.vi"("Chemical Name"=w361) -> ("error out"=w364:errorcluster, "Downloaded Picture"=w365:picture)  [unwired: 8 in, 1 out]
                                n141 = Unbundle By Name(w364) -> ("status"=w359:bool)
                                n142 = Not(x=w359) -> (.not. x?=w360:bool)
                                n143 = case shown="False" w360 {
                                tunnel: w365 -> [_ w368]
                                tunnel: [w366 w367] -> w362
                                tunnel: w363 -> [w366 _]
                                frame False {
                                }
                                frame True {
                                n144 = call <vilib>:"Draw Flattened Pixmap.vi"("picture"=w368) -> ("new picture"=w367:picture)  [unwired: 8 in]
                                }
                                }
                                }
                                }
                                n145 = local write "Reagent Pic 4"(w353) -> ()
                              }
                              frame #1 {
                                n146 = Wait (ms)(milliseconds to wait=100) -> ()  [unwired: 1 out]
                              }
                            }
                          }
                          frame #6 {
                            n147 = flat-sequence {
                              tunnel: w371 -> [w375]
                              tunnel: w370 -> [w374]
                              frame #0 {
                                n148 = local read "reagent  name 3"() -> (w372:string)
                                n149 = String Length(string=w372) -> (length=w377:i32)
                                n150 = Greater Than 0?(x=w377) -> (x > 0?=w376:bool)
                                n151 = case shown="True" w376 {
                                tunnel: w374 -> [_ w383]
                                tunnel: w375 -> [w378 _]
                                tunnel: [w378 w382] -> w373
                                tunnel: w372 -> [_ w381]
                                frame False {
                                }
                                frame True {
                                n152 = call "Image_from_name.vi"("Chemical Name"=w381) -> ("error out"=w384:errorcluster, "Downloaded Picture"=w385:picture)  [unwired: 8 in, 1 out]
                                n153 = Unbundle By Name(w384) -> ("status"=w379:bool)
                                n154 = Not(x=w379) -> (.not. x?=w380:bool)
                                n155 = case shown="False" w380 {
                                tunnel: w385 -> [_ w388]
                                tunnel: [w386 w387] -> w382
                                tunnel: w383 -> [w386 _]
                                frame False {
                                }
                                frame True {
                                n156 = call <vilib>:"Draw Flattened Pixmap.vi"("picture"=w388) -> ("new picture"=w387:picture)  [unwired: 8 in]
                                }
                                }
                                }
                                }
                                n157 = local write "Reagent Pic 3"(w373) -> ()
                              }
                              frame #1 {
                                n158 = Wait (ms)(milliseconds to wait=100) -> ()  [unwired: 1 out]
                              }
                            }
                          }
                        }
                      }
                      frame #3 {
                        n159 = local read "BAY 1"() -> (w400:u16)
                        n160 = local read "BAY 2"() -> (w399:u16)
                        n161 = local read "BAY 3"() -> (w398:u16)
                        n162 = local read "BAY 4"() -> (w397:u16)
                        n163 = local read "BAY 5"() -> (w396:u16)
                        n164 = local read "tube_id(in)"() -> (w407:enum16{".01", ".02", ".03", ".04"}[])
                        n165 = local read "Vr4"() -> (w410:dbl)
                        n166 = local read "tube_length(in)"() -> (w408:dbl[])
                        n167 = Build Array(w400, w399, w398, w397, w396) -> (w395:u16[])
                        n168 = local read "Vr3"() -> (w411:dbl)
                        n169 = local read "new_reactor_length"() -> (w405:bool[])
                        n170 = local read "Vr1"() -> (w413:dbl)
                        n171 = local read "Vr5"() -> (w409:dbl)
                        n172 = local read "Vr2"() -> (w412:dbl)
                        n173 = local read "new_reactor_volume"() -> (w403:bool[])
                        n174 = for {
                          N: 5 -> [_]
                          tunnel: w403 -> [w417] mode=indexing
                          tunnel: [w414] -> w401 mode=indexing
                          n175 = Select(t=1.0, s=w417, f=0.0) -> (s? t:f=w414:dbl)
                        }
                        n176 = for {
                          N: 5 -> [_]
                          tunnel: w405 -> [w421] mode=indexing
                          tunnel: [w418] -> w404 mode=indexing
                          n177 = Select(t=1.0, s=w421, f=0.0) -> (s? t:f=w418:dbl)
                        }
                        n178 = script code="tube_diameters = [.01,.02,.03,.04];\naddpath('C:\\Users\\HPLC\\Dropbox (MIT)\\MoD Files\\MATLAB');\ncalculate_reactor_volumes;"("BayConfig"=w395, "Vr1"=w413, "Vr2"=w412, "Vr3"=w411, "Vr4"=w410, "Vr5"=w409, "tube_length"=w408, "tube_id"=w407, "new_len_react"=w404, "new_vol_react"=w401) -> ("Vr1"=w394:dbl, "Vr2"=w393:dbl, "Vr3"=w392:dbl, "Vr4"=w391:dbl, "Vr5"=w390:dbl)  [unwired: 1 in, 1 out]
                        n179 = local write "Vr1"(w394) -> ()
                        n180 = local write "Vr2"(w393) -> ()
                        n181 = local write "Vr3"(w392) -> ()
                        n182 = local write "Vr4"(w391) -> ()
                        n183 = local write "Vr5"(w390) -> ()
                      }
                      frame #4 {
                        n184 = local read "Setup Error"() -> (w424:bool)
                        n185 = case shown="True" w424 {
                          tunnel: [TRUE FALSE] -> w422
                          tunnel: ["" "Sytem setup has not been confirmed!"] -> w423
                          frame False {
                          }
                          frame True {
                            n186 = local read "Error Message"() -> (w429:string)
                            n187 = One Button Dialog(message=w429) -> ()  [unwired: 1 in, 1 out]
                          }
                        }
                        n188 = local write "System Confirm Not Clicked"(w423) -> ()
                        n189 = local write "Setup Confirm"(w422) -> ()
                      }
                    }
                  }
                }
              }
            }
            n190 = local read "Stop"() -> (w208:bool)
            n191 = Or(x=w209, y=w208) -> (x .or. y?=w207:bool)
            n192 = disable-structure shown="Disabled" {
              disable-tunnel: 400 -> [w215 _]
              frame Disabled {
                n193 = event shown="[1]" {
                  selector: _ -> [_ _]
                  dyn-events: _ -> [_ _]
                  timeout: w215 -> [_ _]
                  event Timeout {
                    n194 = event-data() -> ()  [unwired: 1 in, 3 out]
                  }
                  event #1 (no event record) {
                    n195 = event-data() -> ()  [unwired: 1 in, 6 out]
                    n196 = local read "Setup Confirm"() -> (w216:bool)
                    n197 = local read "Reaction Scheme Confirm"() -> (w217:bool)
                    n198 = Not(x=w216) -> (.not. x?=w219:bool)
                    n199 = And(x=w217, y=w219) -> (x .and. y?=w218:bool)
                    n200 = case shown="True" w218 {
                      frame False {
                      }
                      frame True {
                        w221 = u16 0 items=["                     Bypass", "                Hot Reactor", "                 Separator"] ("BAY 5")
                        w222 = u16 0 items=["                     Bypass", "                Hot Reactor", "                  Separator"] ("BAY 4")
                        w223 = u16 0 items=["                     Bypass", "                 Hot Reactor", "                  Separator"] ("BAY 3")
                        w224 = u16 0 items=["                     Bypass", "                Hot Reactor", "                  Separator"] ("BAY 2")
                        w225 = u16 0 items=["                 Bypass", "             Hot Reactor", "               Separator"] ("BAY 1")
                        n201 = local write "BAY 3"(w223) -> ()
                        n202 = local write "BAY 4"(w222) -> ()
                        n203 = local write "BAY 5"(w221) -> ()
                        n204 = local write "BAY 2"(w224) -> ()
                        n205 = local write "BAY 1"(w225) -> ()
                        n206 = local write "Synthesis Route Array"(string[][] [["3-Br-Pyridine _ Biphenyl", "K2CO3", "PhB(OH)2", "", "", ""]] ("Synthesis Route Array")) -> ()
                      }
                    }
                  }
                }
              }
              frame Enabled {
              }
            }
            n207 = disable-structure shown="Disabled" {
              disable-tunnel: 400 -> [w211 _]
              frame Disabled {
                n208 = event shown="[1]" {
                  selector: _ -> [_ _]
                  dyn-events: _ -> [_ _]
                  timeout: w211 -> [_ _]
                  event Timeout {
                    n209 = event-data() -> ()  [unwired: 1 in, 3 out]
                  }
                  event #1 (no event record) {
                    n210 = event-data() -> ()  [unwired: 1 in, 6 out]
                    n211 = call "File Dialog"("prompt"="Load previously saved xml file") -> ("selected path"=w213:path)  [unwired: 11 in, 3 out]
                    n212 = Path To String(path=w213) -> (string=w212:string)
                    n213 = script code="xmlDoc = xmlread(file_path);\nroot = xmlDoc.getDocumentElement();\nb = root.getChildNodes;\nrecipe = b.getElementsByTagName('Bay1').item(0);"("file_path"=w212) -> ()  [unwired: 1 in, 1 out]
                  }
                }
              }
              frame Enabled {
              }
            }
          }
        }
        frame #1 {
          n214 = local read "Stop"() -> (w431:bool)
          n215 = Not(x=w431) -> (.not. x?=w430:bool)
          n216 = case shown="True" w430 {
            tunnel: w432 -> [_ w435]
            frame False {
              "stop_button clicked" <- TRUE ("stop_button clicked")
            }
            frame True {
              # "Parameters Initilization"
              n217 = flat-sequence {
                tunnel: w435 -> [w437]
                tunnel: [w436] -> w434
                tunnel: w434 -> [w596]
                frame #0 {
                  # "Setup bays(RFID - verify)"
                  n218 = disable-structure shown="Disabled" {
                    frame Disabled {
                      n219 = local read "BAY 1"() -> ()  [unwired: 1 out]
                      n220 = local read "BAY 2"() -> ()  [unwired: 1 out]
                      n221 = local read "BAY 3"() -> ()  [unwired: 1 out]
                      n222 = local read "BAY 4"() -> ()  [unwired: 1 out]
                      n223 = local read "BAY 5"() -> ()  [unwired: 1 out]
                    }
                    frame Enabled {
                    }
                  }
                }
                frame #1 {
                  n224 = while {
                    tunnel: w437 -> [w440]
                    tunnel: [w439] -> w436
                    stop <- w443 stop-if-true
                    n225 = flat-sequence {
                      tunnel: [w457] -> w439
                      tunnel: w440 -> [w538]
                      tunnel: [w456] -> w438
                      frame #0 {
                        n226 = while {
                          stop <- w447 stop-if-true
                          n227 = event shown="[1] \"System Parameters Confirm Button\": Value Change" {
                            selector: _ -> [_ _]
                            dyn-events: _ -> [_ _]
                            timeout: u32 200 ("milliseconds to wait") -> [_ _]
                            tunnel: [FALSE TRUE] -> w445
                            event Timeout {
                              n228 = event-data() -> ()  [unwired: 1 in, 3 out]
                            }
                            event "System Parameters Confirm Button": Value Change {
                              n229 = event-data() -> ()  [unwired: 1 in, 5 out]
                              n230 = local write "System Parameters Confirm Button"(FALSE) -> ()
                            }
                          }
                          n231 = Wait (ms)(milliseconds to wait=u32 500) -> ()  [unwired: 1 out]
                          n232 = local read "Stop"() -> (w448:bool)
                          n233 = Or(x=w448, y=w445) -> (x .or. y?=w447:bool)
                        }
                      }
                      frame #1 {
                        w477 = 0 ("disabled index (col)")
                        w489 = 1 ("disabled index (col)")
                        # "Do while parameters have not been correctly entered"
                        n234 = local read "Bay Parameters"() -> (w476:T2)
                        n235 = local read "Synthesis Route Array"() -> (w490:string[][])
                        n236 = local read "Total Number of Experiments"() -> (w509:dbl)
                        n237 = Unbundle By Name(w476) -> ("Continue from previous optimization?"=w537:bool)
                        n238 = Unbundle By Name(w476) -> ("Excel File Name"=w539:string)
                        n239 = Unbundle By Name(w476) -> ("Matlab File"=w535:string)
                        n240 = Unbundle By Name(w476) -> ("Bay 1.Run at set flowrate"=w581:bool)
                        n241 = Unbundle By Name(w476) -> ("Bay 1.Pump 1 Flowrate"=w587:dbl)
                        n242 = Unbundle By Name(w476) -> ("Bay 1.Pump 2 Flowrate"=w586:dbl)
                        n243 = Unbundle By Name(w476) -> ("Bay 2.Run at set flowrate"=w579:bool)
                        n244 = Unbundle By Name(w476) -> ("Bay 2.Pump 3 Flowrate"=w585:dbl)
                        n245 = Unbundle By Name(w476) -> ("Bay 3.Pump 4 Flowrate"=w584:dbl)
                        n246 = Unbundle By Name(w476) -> ("Bay 3.Run at set flowrate"=w578:bool)
                        n247 = Unbundle By Name(w476) -> ("Bay 4.Run at set flowrate"=w575:bool)
                        n248 = Unbundle By Name(w476) -> ("Bay 4.Pump 5 Flowrate"=w583:dbl)
                        n249 = Unbundle By Name(w476) -> ("Bay 5.Pump 6 Flowrate"=w582:dbl)
                        n250 = Unbundle By Name(w476) -> ("Bay 5.Run at set flowrate"=w574:bool)
                        n251 = Index Array(array=w490, index (row)=3, index (col)=w489) -> (element=w483:string)
                        n252 = Index Array(array=w490, index (row)=2, index (col)=w489) -> (element=w481:string)
                        n253 = Index Array(array=w490, index (row)=1, index (col)=w489) -> (element=w479:string)
                        n254 = Index Array(array=w490, index (row)=0, index (col)=w489) -> (element=w492:string)
                        n255 = Index Array(array=w490, index (row)=4, index (col)=w489) -> (element=w485:string)
                        n256 = Index Array(array=w490, index (row)=5, index (col)=w489) -> (element=w487:string)
                        n257 = Build Array(w492, w479, w481, w483, w485, w487) -> (w493:string[])
                        n258 = Index Array(array=w490, index (row)=0 ("index"), index (col)=w477) -> (element=w515:string)
                        n259 = for {
                          tunnel: w493 -> [w589] mode=indexing
                          tunnel: [w588] -> w478 mode=indexing
                          n260 = script code="ctemp1 = str2num(c_temp);"("c_temp"=w589) -> ("ctemp1"=w588:dbl)  [unwired: 1 in, 1 out]
                        }
                        n261 = Boolean To (0,1)(Boolean=w579) -> (0, 1=w534:i16)
                        n262 = Boolean To (0,1)(Boolean=w575) -> (0, 1=w576:i16)
                        n263 = Boolean To (0,1)(Boolean=w578) -> (0, 1=w577:i16)
                        n264 = Boolean To (0,1)(Boolean=w537) -> (0, 1=w536:i16)
                        n265 = Boolean To (0,1)(Boolean=w581) -> (0, 1=w580:i16)
                        n266 = Boolean To (0,1)(Boolean=w574) -> (0, 1=w573:i16)
                        n267 = Index Array(array=w490, index (row)=1 ("index"), index (col)=w477) -> (element=w510:string)
                        n268 = Index Array(array=w490, index (row)=2 ("index"), index (col)=w477) -> (element=w511:string)
                        n269 = Unbundle By Name(w476) -> ("Bay 1.optimize_temp"=w572:bool)
                        n270 = Unbundle By Name(w476) -> ("Bay 1.optimize_tau"=w570:bool)
                        n271 = Unbundle By Name(w476) -> ("Bay 2.optimize_temp"=w568:bool)
                        n272 = Unbundle By Name(w476) -> ("Bay 2.optimize_tau"=w566:bool)
                        n273 = Unbundle By Name(w476) -> ("Bay 3.optimize_temp"=w564:bool)
                        n274 = Unbundle By Name(w476) -> ("Bay 3.optimize_tau"=w562:bool)
                        n275 = Unbundle By Name(w476) -> ("Bay 4.optimize_temp"=w560:bool)
                        n276 = Unbundle By Name(w476) -> ("Bay 4.optimize_tau"=w558:bool)
                        n277 = Index Array(array=w490, index (row)=3 ("index"), index (col)=w477) -> (element=w512:string)
                        n278 = Boolean To (0,1)(Boolean=w560) -> (0, 1=w559:i16)
                        n279 = Boolean To (0,1)(Boolean=w558) -> (0, 1=w557:i16)
                        n280 = Index Array(array=w490, index (row)=4 ("index"), index (col)=w477) -> (element=w513:string)
                        n281 = Boolean To (0,1)(Boolean=w562) -> (0, 1=w561:i16)
                        n282 = Boolean To (0,1)(Boolean=w568) -> (0, 1=w567:i16)
                        n283 = Boolean To (0,1)(Boolean=w572) -> (0, 1=w571:i16)
                        n284 = Boolean To (0,1)(Boolean=w566) -> (0, 1=w565:i16)
                        n285 = Boolean To (0,1)(Boolean=w570) -> (0, 1=w569:i16)
                        n286 = Boolean To (0,1)(Boolean=w564) -> (0, 1=w563:i16)
                        n287 = Unbundle By Name(w476) -> ("Bay 5.optimize_temp"=w556:bool)
                        n288 = Unbundle By Name(w476) -> ("Bay 5.optimize_tau"=w554:bool)
                        n289 = Index Array(array=w490, index (row)=5 ("index"), index (col)=w477) -> (element=w514:string)
                        n290 = Boolean To (0,1)(Boolean=w556) -> (0, 1=w555:i16)
                        n291 = Boolean To (0,1)(Boolean=w554) -> (0, 1=w553:i16)
                        n292 = Build Array(w571, w569, w567, w565, w563, w561, w559, w557, w555, w553) -> (w552:i16[])
                        n293 = Unbundle By Name(w476) -> ("Bay 1.Temperature Params"=w549:dbl[])
                        n294 = Unbundle By Name(w476) -> ("Bay 2.Temperature Params"=w548:dbl[])
                        n295 = Unbundle By Name(w476) -> ("Bay 2.Resisdence time params"=w543:dbl[])
                        n296 = Unbundle By Name(w476) -> ("Bay 3.Temperature Params"=w547:dbl[])
                        n297 = Unbundle By Name(w476) -> ("Bay 3.Resisdence time params"=w542:dbl[])
                        n298 = Unbundle By Name(w476) -> ("Bay 4.Temperature Params"=w546:dbl[])
                        n299 = Unbundle By Name(w476) -> ("Bay 4.Resisdence time params"=w541:dbl[])
                        n300 = Unbundle By Name(w476) -> ("Bay 5.Temperature Params"=w545:dbl[])
                        n301 = Unbundle By Name(w476) -> ("Bay 5.Resisdence time params"=w540:dbl[])
                        n302 = Unbundle By Name(w476) -> ("Bay 1.pump params 2"=w508:dbl[])
                        n303 = Unbundle By Name(w476) -> ("Bay 1.pump params 1"=w544:dbl[])
                        n304 = Unbundle By Name(w476) -> ("Bay 1.Run at set temperature"=w499:bool)
                        n305 = Unbundle By Name(w476) -> ("Bay 2.Run at set temperature"=w497:bool)
                        n306 = Unbundle By Name(w476) -> ("Bay 3.Run at set temperature"=w496:bool)
                        n307 = Unbundle By Name(w476) -> ("Bay 4.Run at set temperature"=w495:bool)
                        n308 = Unbundle By Name(w476) -> ("Bay 5.Run at set temperature"=w494:bool)
                        n309 = Unbundle By Name(w476) -> ("Bay 3.Temperature"=w505:dbl)
                        n310 = Unbundle By Name(w476) -> ("Bay 1.Temperature"=w507:dbl)
                        n311 = Unbundle By Name(w476) -> ("Bay 2.Temperature"=w506:dbl)
                        n312 = Unbundle By Name(w476) -> ("Bay 4.Temperature"=w504:dbl)
                        n313 = Unbundle By Name(w476) -> ("Bay 5.Temperature"=w503:dbl)
                        n314 = Unbundle By Name(w476) -> ("Bay 3.pump_num_ratio"=w528:dbl)
                        n315 = Unbundle By Name(w476) -> ("Bay 4.pump_num_ratio"=w525:dbl)
                        n316 = Unbundle By Name(w476) -> ("Bay 5.pump_num_ratio"=w522:dbl)
                        n317 = Unbundle By Name(w476) -> ("Bay 2.pump_num_ratio"=w531:dbl)
                        n318 = Unbundle By Name(w476) -> ("Bay 4.pump_at_ratio"=w527:bool)
                        n319 = Boolean To (0,1)(Boolean=w527) -> (0, 1=w526:i16)
                        n320 = Unbundle By Name(w476) -> ("Bay 3.pump_at_ratio"=w530:bool)
                        n321 = Boolean To (0,1)(Boolean=w530) -> (0, 1=w529:i16)
                        n322 = Unbundle By Name(w476) -> ("Bay 5.pump_at_ratio"=w524:bool)
                        n323 = Boolean To (0,1)(Boolean=w524) -> (0, 1=w523:i16)
                        n324 = Unbundle By Name(w476) -> ("Bay 2.pump_at_ratio"=w533:bool)
                        n325 = Boolean To (0,1)(Boolean=w533) -> (0, 1=w532:i16)
                        n326 = Build Array(w507, w506, w505, w504, w503) -> (w502:dbl[])
                        n327 = Build Array(w499, w497, w496, w495, w494) -> (w498:bool[])
                        n328 = local read "Syringe_pump?"() -> (w455:bool)
                        n329 = for {
                          N: 5 -> [_]
                          tunnel: w498 -> [w593] mode=indexing
                          tunnel: [w592] -> w500 mode=indexing
                          n330 = Select(t=1.0, s=w593, f=0.0) -> (s? t:f=w592:dbl)
                        }
                        n331 = Unbundle By Name(w476) -> ("Internal Standard?"=w467:bool)
                        n332 = Unbundle By Name(w476) -> ("increas_decrease_hplc_peak"=w468:bool)
                        n333 = Unbundle By Name(w476) -> ("Hplc Wait time(min)"=w460:dbl)
                        n334 = Unbundle By Name(w476) -> ("Total Number of Experiments 2"=w459:dbl)
                        n335 = Unbundle By Name(w476) -> ("hplc_start"=w464:dbl)
                        n336 = Unbundle By Name(w476) -> ("ISTD start"=w462:dbl)
                        n337 = Unbundle By Name(w476) -> ("hplc_end"=w463:dbl)
                        n338 = Unbundle By Name(w476) -> ("throughput_yield"=w469:bool)
                        n339 = Unbundle By Name(w476) -> ("ISTD end"=w461:dbl)
                        n340 = Select(t=1.0, s=w455, f=0.0) -> (s? t:f=w454:dbl)
                        n341 = Select(t=1.0, s=w468, f=0.0) -> (s? t:f=w466:dbl)
                        n342 = Select(t=1.0, s=w467, f=0.0) -> (s? t:f=w465:dbl)
                        n343 = Select(t=0.0, s=w469, f=1.0) -> (s? t:f=w458:dbl)
                        n344 = script code="system_error = 0;\nnumPeaks = 1;\nstart_phase_time = 1;\nis_redo_exp = 0;\nfbest_prev = 0;\nxbest_prev = [];\nFvalues = [];\nHPLC_Area = [];\n\nhplc_peak_start3 = 3.21;\nhplc_peak_start2 = 1.8;\n\nhplc_peak_end3 = 4.2;\nhplc_peak_end2 = 2;\n\nT1_span = [1 1]; T2_span = [1 1]; T3_span = [1 1]; T4_span = [1 1]; T5_span = [1 1];\nT_span = [T1_span;T2_span;T3_span;T4_span;T5_span];\n p1_span =  [1 1]; p2_span =  [1 1]; p3_span =  [1 1]; p4_span =  [1 1]; p5_span =  [1 1];  p6_span =  [1 1];\nOpt_params = [0 0 0 0 0 0 0 0 0 0 0];\nT_params = [T1_params;T2_params;T3_params;T4_params;T5_params];\npump_params = [pump1_params;pump2_params;pump3_params;pump4_params;pump5_params;pump6_params];\nopt_ctr = 0;ncall = 100;record_data = true;\nT1_SP = 23; T2_SP = 23; T3_SP = 23; T4_SP = 23; T5_SP = 23;\nT_span = [T1_span;T2_span;T3_span;T4_span;T5_span];\np_span = [p1_span;p2_span;p3_span;p4_span;p5_span;p6_span];\nno_errors = 1;\nP1 = 0; P2 =0; P3 = 0; P4 = 0; P5 = 0; P6 = 0;\nP = [P1, P2, P3,P4, P5, P6];\nis_first_set_of_exp = true;\nerror_message = 'System has no errors to report';\naddpath(genpath('C:\\Users\\HPLC\\Dropbox (MIT)\\MoD Files\\MATLAB'))\n%addpath(genpath('C:\\Users\\Admin\\Dropbox (MIT)\\MoD Files\\MATLAB'))\nallMSData = [];allHPLCData = [];allHPLCFile = [];\nBay_ratio = [0,Bay2_ratio,Bay3_ratio,Bay4_ratio,Bay5_ratio];\nBay_pump_ratio = [1, Bay2_pump_ratio, Bay3_pump_ratio, Bay4_pump_ratio, Bay5_pump_ratio];\nP_setrate = [P1_setrate, P2_setrate, P3_setrate, P4_setrate, P5_setrate, P6_setrate];\nuse_flowrate = [use_flowrate1, use_flowrate2,use_flowrate3, use_flowrate4, use_flowrate5];\npump_chem_name= []\nCurrExp = 1;\n% ****************************************************************************************************\n%Setup optimization\n   setup_optimization_params;\n   initialize_opt = 0;\n   nstop0 = 0;\n%*****************************************************************************************************\n% Setup excel and xml file writing\npath(path, pa);\nnumMSSig = 1;\nsetup_excel_output;\n%***************************************************************************************************\nredo = false;\nncall = ncall_in;"("use_flowrate1"=w580, "P1_setrate"=w587, "P2_setrate"=w586, "P3_setrate"=w585, "P4_setrate"=w584, "P5_setrate"=w583, "P6_setrate"=w582, "use_flowrate2"=w534, "use_flowrate3"=w577, "use_flowrate4"=w576, "use_flowrate5"=w573, "Optimize_params"=w552, "T1_params"=w549, "T2_params"=w548, "T3_params"=w547, "T4_params"=w546, "T5_params"=w545, "pump1_params"=w544, "pump3_params"=w543, "pump4_params"=w542, "pump5_params"=w541, "pump6_params"=w540, "xl_file"=w539, "pa"=w538, "Continue"=w536, "matlabsavefile"=w535, "Bay2_ratio"=w532, "Bay2_pump_ratio"=w531, "Bay3_ratio"=w529, "Bay3_pump_ratio"=w528, "Bay4_ratio"=w526, "Bay4_pump_ratio"=w525, "Bay5_ratio"=w523, "Bay5_pump_ratio"=w522, "pump1_chem"=w515, "pump6_chem"=w514, "pump5_chem"=w513, "pump4_chem"=w512, "pump3_chem"=w511, "pump2_chem"=w510, "Pump_concen"=w478, "ncall_in"=w509, "pump2_params"=w508, "T_SP"=w502, "Run_at_T_SP"=w500, "dcr_hplc_peak"=w466, "use_internal_std"=w465, "hplc_peak_start"=w464, "hplc_peak_end"=w463, "ISTD_start"=w462, "ISTD_end"=w461, "hplc_wait_time"=w460, "tot_num_exp"=w459, "throughput_yield"=w458, "syringe_pump"=w454) -> ("no_errors"=w551:dbl, "error_message"=w550:string)  [unwired: 1 in, 1 out]
                        n345 = Not Equal To 0?(x=w551) -> (x != 0?=w456:bool)
                        n346 = Not(x=w456) -> (.not. x?=w457:bool)
                        n347 = case shown="False" w457 {
                          tunnel: w550 -> [_ w595]
                          frame False {
                            n348 = local write "Setup Confirm 2"(TRUE ("Setup Confirm 2")) -> ()
                          }
                          frame True {
                            n349 = One Button Dialog(message=w595) -> ()  [unwired: 1 in, 1 out]
                          }
                        }
                      }
                    }
                    n350 = local read "Stop"() -> (w442:bool)
                    n351 = Or(x=w438, y=w442) -> (x .or. y?=w443:bool)
                    n352 = Wait (ms)(milliseconds to wait=u32 500) -> ()  [unwired: 1 out]
                  }
                }
                frame #2 {
                  n353 = local write "System Error"(w596) -> ()
                }
              }
            }
          }
        }
        frame #2 {
          # "Run Initial diagnostics"
        }
        frame #3 {
          # "Run System"
          n354 = while {
            tunnel: w597 -> [w1358]
            stop <- w1362 stop-if-true
            n355 = local read "running?"() -> (w1357:bool)
            n356 = local read "Temperature Control 1"() -> (w1359:bool)
            n357 = And(x=w1357, y=w1359) -> (x .and. y?=w1360:bool)
            n358 = case shown="False" w1360 {
              tunnel: w1358 -> [_ w1364]
              frame False {
                n359 = local write "Temp SS? 1"(TRUE ("Temp SS? 1")) -> ()
              }
              frame True {
                # "Bay 1 Temperature Controller"
                n360 = local read "Temperature SP 1"() -> (w1365:dbl)
                n361 = local read "Temperature 1"() -> (w1369:dbl)
                n362 = local read "SSR Duration 1"() -> (w1384:dbl)
                n363 = call-poly <vilib>:"PID Online Autotuning.vi"("setpoint"=w1365, "manipulated variable"=w1384, "autotuning parameters"=T9 {"type of controller"=enum."PID", "relay cycles"=3, "relay amplitude"=1.0, "control specifications"=enum."Normal", "PV noise level"=0.1} ("Autotuning Parameters R1"), "process variable"=w1369, "PID gains in"=T8 {"Proportional gain Kc"=0.38538, "Integral time Ti (sec)"=0.524375, "Derivative time Ti (sec)"=0.12585} ("PID gains 2")) -> ("setpoint out"=w1390:dbl, "process variable out"=w1389:dbl, "PID gains out"=w1386:T17)  [unwired: 6 in, 2 out]
                n364 = call <vilib>:"PID Autotuning (Temperature).vi"("desired temperature"=w1390, "measured temperature"=w1389, "plant parameters in"=w1386, "output range"=cluster{"output high":dbl, "output low":dbl} {"output high"=3.0, "output low"=-1.0} ("Output range")) -> ("output"=w1382:dbl)  [unwired: 12 in, 3 out]
                n365 = local write "SSR Duration 1"(w1382) -> ()
                n366 = Subtract(x=w1365, y=w1369) -> (x-y=w1376:dbl)
                n367 = Absolute Value(x=w1376) -> (abs(x)=w1379:dbl)
                n368 = Multiply(x=1000.0, y=w1382) -> (x*y=w1380:dbl)
                n369 = Greater Than 0?(x=w1380) -> (x > 0?=w1374:bool)
                n370 = Less Or Equal?(x=w1379, y=1.2) -> (x <= y?=w1377:bool)
                n371 = Greater?(x=w1365, y=w1369) -> (0:w1375:bool)
                n372 = And(x=w1374, y=w1375) -> (x .and. y?=w1372:bool)
                n373 = local write "Temp SS? 1"(w1377) -> ()
                n374 = Subtract(x=w1369, y=10.0) -> (x-y=w1370:dbl)
                n375 = Less?(x=w1370, y=w1365) -> (x < y?=w1373:bool)
                n376 = And(x=w1373, y=w1372) -> (x .and. y?=w1371:bool)
                n377 = case shown="True" w1371 {
                  tunnel: [errorcluster {"status"=FALSE, "code"=0, "source"=""} ("error out") w1400] -> _
                  tunnel: 2 -> [_ w1397]
                  tunnel: w1380 -> [w1394 w1398]
                  tunnel: [0.0 w1402] -> w1367
                  tunnel: w1365 -> [_ w1401]
                  tunnel: w1364 -> [_ w1399]
                  frame False {
                    n378 = Absolute Value(x=w1394) -> (abs(x)=w1395:dbl)
                    n379 = Wait (ms)(milliseconds to wait=w1395) -> ()  [unwired: 1 out]
                  }
                  frame True {
                    n380 = call "TurnOnRelayArduino.vi"("channel"=w1397, "duration"=w1398, "LINX Resource"=w1399) -> ("error out"=w1400:errorcluster)  [unwired: 7 in, 1 out]
                    n381 = script code="tempdiff1= SP1 - T1;\nif tempdiff1 > 10\n  if slope1 < .01\n     temp_check1 = temp_check1 + 1;\n  else\n      temp_check1 =0;\n  end\nend\n\nif temp_check1 > 9\n  temp_error1 = 1\nend"("SP1"=w1401) -> ("temp_error1"=w1402:dbl)  [unwired: 1 in, 1 out]
                  }
                }
                n382 = Not Equal To 0?(x=w1367) -> (x != 0?=w1366:bool)
                n383 = case shown="True" w1366 {
                  frame False {
                  }
                  frame True {
                    n384 = local write "Error Message"("Bay 1 Temperature Heating Error") -> ()
                  }
                }
                n385 = case shown="True" w1366 {
                  tunnel: w1366 -> [_ w1392]
                  frame False {
                  }
                  frame True {
                    n386 = local write "System Error"(w1392) -> ()
                    n387 = local write "Stop"(w1392) -> ()
                  }
                }
              }
            }
            n388 = Wait (ms)(milliseconds to wait=u32 400) -> ()  [unwired: 1 out]
            n389 = local read "Stop"() -> (w1362:bool)
          }
          n390 = local read "Bay Parameters"() -> (w601:T2)
          n391 = while {
            tunnel: w597 -> [w1311]
            stop <- w1315 stop-if-true
            n392 = local read "Temperature Control 2"() -> (w1312:bool)
            n393 = local read "running?"() -> (w1310:bool)
            n394 = And(x=w1310, y=w1312) -> (x .and. y?=w1313:bool)
            n395 = case shown="True" w1313 {
              tunnel: w1311 -> [_ w1318]
              frame False {
                n396 = flat-sequence {
                  frame #0 {
                    n397 = local write "Temp SS? 2"(TRUE ("Temp SS? 2")) -> ()
                  }
                  frame #1 {
                    n398 = local read "Temp SS? 2"() -> (→"Temp SS? 6":bool)
                  }
                }
              }
              frame True {
                # "Bay 2 Temperature Controller"
                n399 = local read "Temperature SP 2"() -> (w1320:dbl)
                n400 = local read "Temperature 2"() -> (w1323:dbl)
                n401 = local read "SSR Duration 2"() -> (w1341:dbl)
                n402 = call-poly <vilib>:"PID Online Autotuning.vi"("setpoint"=w1320, "manipulated variable"=w1341, "autotuning parameters"=T9 {"type of controller"=enum."PID", "relay cycles"=3, "relay amplitude"=1.0, "control specifications"=enum."Normal", "PV noise level"=0.1} ("Autotuning Parameters R1"), "process variable"=w1323, "PID gains in"=T8 {"Proportional gain Kc"=0.38538, "Integral time Ti (sec)"=0.524375, "Derivative time Ti (sec)"=0.12585} ("PID gains 2")) -> ("setpoint out"=w1339:dbl, "process variable out"=w1338:dbl, "PID gains out"=w1344:T17)  [unwired: 6 in, 2 out]
                n403 = call <vilib>:"PID Autotuning (Temperature).vi"("desired temperature"=w1339, "measured temperature"=w1338, "plant parameters in"=w1344, "output range"=cluster{"output high":dbl, "output low":dbl} {"output high"=3.0, "output low"=-1.0} ("Output range")) -> ("output"=w1334:dbl)  [unwired: 12 in, 3 out]
                n404 = local write "SSR Duration 2"(w1334) -> ()
                n405 = Greater?(x=w1320, y=w1323) -> (0:w1329:bool)
                n406 = Multiply(x=1000.0, y=w1334) -> (x*y=w1336:dbl)
                n407 = Greater Than 0?(x=w1336) -> (x > 0?=w1328:bool)
                n408 = And(x=w1328, y=w1329) -> (x .and. y?=w1326:bool)
                n409 = Subtract(x=w1320, y=w1323) -> (x-y=w1331:dbl)
                n410 = Absolute Value(x=w1331) -> (abs(x)=w1333:dbl)
                n411 = Subtract(x=w1323, y=10.0) -> (x-y=w1325:dbl)
                n412 = Less Or Equal?(x=w1333, y=1.2) -> (x <= y?=w1330:bool)
                n413 = local write "Temp SS? 2"(w1330) -> ()
                n414 = Less?(x=w1325, y=w1320) -> (x < y?=w1327:bool)
                n415 = And(x=w1327, y=w1326) -> (x .and. y?=w1322:bool)
                n416 = case shown="True" w1322 {
                  tunnel: [errorcluster {"status"=FALSE, "code"=0, "source"=""} ("error out") w1354] -> _
                  tunnel: 3 -> [_ w1351]
                  tunnel: w1336 -> [w1348 w1352]
                  tunnel: [0.0 w1356] -> w1321
                  tunnel: w1320 -> [_ w1355]
                  tunnel: w1318 -> [_ w1353]
                  frame False {
                    n417 = Absolute Value(x=w1348) -> (abs(x)=w1349:dbl)
                    n418 = Wait (ms)(milliseconds to wait=w1349) -> ()  [unwired: 1 out]
                  }
                  frame True {
                    n419 = call "TurnOnRelayArduino.vi"("channel"=w1351, "duration"=w1352, "LINX Resource"=w1353) -> ("error out"=w1354:errorcluster)  [unwired: 7 in, 1 out]
                    n420 = script code="tempdiff2= SP2 - T2;\nif tempdiff2 > 10\n  if slope2 < .01\n     temp_check2 = temp_check2 + 1;\n  else\n      temp_check2 =0;\n  end\nend\n\nif temp_check2 > 9\n  temp_error2 = 1\nend"("SP2"=w1355) -> ("temp_error2"=w1356:dbl)  [unwired: 1 in, 1 out]
                  }
                }
                n421 = Not Equal To 0?(x=w1321) -> (x != 0?=w1319:bool)
                n422 = case shown="True" w1319 {
                  frame False {
                  }
                  frame True {
                    n423 = local write "Error Message"("Bay 2 Temperature Heating Error") -> ()
                  }
                }
                n424 = case shown="True" w1319 {
                  tunnel: w1319 -> [_ w1346]
                  frame False {
                  }
                  frame True {
                    n425 = local write "Stop"(w1346) -> ()
                    n426 = local write "System Error"(w1346) -> ()
                  }
                }
              }
            }
            n427 = local read "Stop"() -> (w1315:bool)
            n428 = Wait (ms)(milliseconds to wait=u32 400) -> ()  [unwired: 1 out]
          }
          n429 = local read "Stop"() -> (w598:bool)
          n430 = Not(x=w598) -> (.not. x?=w600:bool)
          n431 = case shown="True" w600 {
            tunnel: w601 -> [_ w606]
            tunnel: w599 -> [_ w605]
            tunnel: w597 -> [_ w604]
            frame False {
            }
            frame True {
              n432 = while {
                tunnel: w606 -> [w620]
                tunnel: w605 -> [w612]
                tunnel: w604 -> [w607]
                i -> [w619]
                stop <- w613 stop-if-true
                n433 = local read "running?"() -> (w608:bool)
                n434 = Wait (ms)(milliseconds to wait=u32 1000) -> ()  [unwired: 1 out]
                n435 = Increment(x=w619) -> (x+1=w609:i32)
                n436 = case shown="True" w608 {
                  tunnel: w619 -> [w625 _]
                  tunnel: w620 -> [_ _]
                  tunnel: [w627 w631] -> w610
                  tunnel: [0.0 w632] -> w615
                  tunnel: w612 -> [_ w630]
                  tunnel: w607 -> [_ w628]
                  frame False {
                    # "STANDBY MODE"
                    n437 = Add(x=w625, y=2.0) -> (x+y=w627:dbl)
                  }
                  frame True {
                    n438 = flat-sequence {
                      tunnel: w630 -> [w634]
                      tunnel: [w634] -> w629
                      tunnel: [w645] -> w632
                      tunnel: [200.0] -> w631
                      tunnel: w629 -> [w643]
                      tunnel: w628 -> [w635]
                      frame #0 {
                        n439 = local write "stop_xl_write"(FALSE ("stop_xl_write")) -> ()
                      }
                      frame #1 {
                        # "Increase flowrate of dilution stream"
                        # "Wait mixed stream reaches SL"
                        # "SNOBFIT"
                        # "Optimize"
                        # "Run Experimental Conditions"
                        # "Optimize/Synthesize"
                        n440 = local read "Syringe_pump?"() -> (w637:bool)
                        n441 = local read "Stop"() -> (w640:bool)
                        n442 = Not(x=w640) -> (.not. x?=w639:bool)
                        n443 = case shown="True" w639 {
                          tunnel: [1.0 w667] -> w648
                          tunnel: [w655 w666] -> w642
                          tunnel: [0.0 w665] -> w641
                          tunnel: [w655 w664] -> w638
                          tunnel: w637 -> [_ w661]
                          frame False {
                            w655 = dbl[] []
                          }
                          frame True {
                            n444 = Select(t=1.0, s=w661, f=0.0) -> (s? t:f=w660:dbl)
                            n445 = script code="optimization_main_loop_ketene"("syringe_pump"=w660) -> ("Conditions_Array"=w666:dbl[], "opt_ctr"=w667:dbl, "P_tot"=w665:dbl, "tau_array"=w664:dbl[], "experiment_history"=w662:dbl[][])  [unwired: 1 in, 1 out]
                            n446 = call-poly <vilib>:"Array To Matrix.vi"("Real 2D Array"=w662) -> ("Real Matrix"=w663:T18)
                            n447 = local write "experiment history"(w663) -> ()
                          }
                        }
                        "P_tot" <- w641
                        n448 = local read "COMM Port :: Milligat Pumps"() -> (w649:refnum<visa-resource-name>)
                        n449 = Equal?(x=w648, y=1.0) -> (x = y?=w646:bool)
                        n450 = flat-sequence {
                          tunnel: w642 -> [w1155]
                          tunnel: w638 -> [w1149]
                          frame #0 {
                            # "Start recording data"
                            n451 = Index Array(array=w1155, index=5) -> (element=w1167:dbl)
                            n452 = Index Array(array=w1155, index=0) -> (element=w1162:dbl)
                            n453 = Index Array(array=w1155, index=1) -> (element=w1163:dbl)
                            n454 = Index Array(array=w1155, index=2) -> (element=w1165:dbl)
                            n455 = Index Array(array=w1155, index=3) -> (element=w1164:dbl)
                            n456 = Index Array(array=w1155, index=4) -> (element=w1166:dbl)
                            n457 = local write "Pump setpoint(ul/min) 2"(w1163) -> ()
                            n458 = local write "Pump setpoint(ul/min) 4"(w1165) -> ()
                            n459 = local write "Pump setpoint(ul/min) 5"(w1166) -> ()
                            n460 = local write "Pump setpoint(ul/min) 3"(w1164) -> ()
                            n461 = local write "Pump setpoint(ul/min) 6"(w1167) -> ()
                            n462 = local write "Pump setpoint(ul/min) 1"(w1162) -> ()
                            n463 = Index Array(array=w1149, index=0) -> (element=w1154:dbl)
                            n464 = Index Array(array=w1149, index=4) -> (element=w1153:dbl)
                            n465 = Index Array(array=w1149, index=3) -> (element=w1152:dbl)
                            n466 = Index Array(array=w1149, index=2) -> (element=w1151:dbl)
                            n467 = Index Array(array=w1149, index=1) -> (element=w1150:dbl)
                            n468 = local write "tau 2"(w1150) -> ()
                            n469 = local write "tau 3"(w1151) -> ()
                            n470 = local write "tau 4"(w1152) -> ()
                            n471 = local write "tau 5"(w1153) -> ()
                            n472 = local write "tau 1"(w1154) -> ()
                          }
                        }
                        n473 = flat-sequence {
                          tunnel: w649 -> [w672]
                          tunnel: w642 -> [w671]
                          tunnel: w646 -> [w670]
                          tunnel: [w670] -> w654
                          tunnel: w643 -> [w669]
                          tunnel: w654 -> [w868]
                          tunnel: [w868] -> w653
                          tunnel: w653 -> [w888]
                          tunnel: [w886] -> w636
                          tunnel: w642 -> [w912]
                          tunnel: w635 -> [w910]
                          tunnel: w635 -> [_]
                          tunnel: w636 -> [w911]
                          tunnel: [w1085] -> w652
                          tunnel: w652 -> [w1098]
                          tunnel: [w1098] -> w651
                          tunnel: w651 -> [w1106]
                          tunnel: [w1106] -> w650
                          tunnel: [w1143] -> w645
                          tunnel: w650 -> [w1143]
                          frame #0 {
                            # "Setup pump flowrates and temperature setpoints"
                            n474 = local read "Pump Addresses"() -> (w668:string[])
                            n475 = stacked-sequence {
                              tunnel: w672 -> [w699 _ _ _ _]
                              tunnel: w672 -> [_ w755 _ _ _]
                              tunnel: w672 -> [_ _ w788 _ _]
                              tunnel: w672 -> [_ _ _ w821 _]
                              tunnel: w672 -> [_ _ _ _ w854]
                              tunnel: w671 -> [w696 w753 w786 w819 w851]
                              tunnel: w670 -> [w688 w748 w781 w814 w847]
                              tunnel: w669 -> [w686 _ _ _ _]
                              tunnel: w668 -> [w678 w740 w768 w806 w839]
                              frame #0 {
                                # "Bay 1"
                                n476 = local read "Syringe_pump?"() -> (w687:bool)
                                n477 = Index Array(array=w696, index=0) -> (element=w694:dbl)
                                n478 = local read "BAY 1"() -> (w681:u16)
                                n479 = Index Array(array=w696, index=1) -> (element=w693:dbl)
                                n480 = Index Array(array=w696, index=6) -> (element=w673:dbl)
                                n481 = script code="MATLAB script"("T1_SP"=w673) -> ()  [unwired: 1 in, 1 out]
                                n482 = Less Or Equal?(x=w681, y=u16 4) -> (x <= y?=w683:bool)
                                n483 = Greater Or Equal?(x=w681, y=u16 1) -> (x >= y?=w684:bool)
                                n484 = And(x=w684, y=w683) -> (x .and. y?=w685:bool)
                                n485 = Greater Than 0?(x=w694) -> (x > 0?=w692:bool)
                                n486 = And(x=w692, y=w688) -> (x .and. y?=w691:bool)
                                n487 = Greater Than 0?(x=w693) -> (x > 0?=w690:bool)
                                n488 = Wait (ms)(milliseconds to wait=u32 300) -> ()  [unwired: 1 out]
                                n489 = And(x=w690, y=w688) -> (x .and. y?=w689:bool)
                                n490 = And(x=w685, y=w688) -> (x .and. y?=w675:bool)
                                n491 = Not Equal?(x=w673, y=23.0) -> (x != y?=w676:bool)
                                n492 = And(x=w675, y=w676) -> (x .and. y?=w674:bool)
                                n493 = case shown="True" w687 {
                                tunnel: w699 -> [w703 _]
                                tunnel: w693 -> [w702 w714]
                                tunnel: w689 -> [w701 w715]
                                tunnel: w686 -> [_ w713]
                                tunnel: w678 -> [w700 _]
                                frame False {
                                n494 = case shown="True" w701 {
                                tunnel: w703 -> [w706 w712]
                                tunnel: w702 -> [_ w711]
                                tunnel: w700 -> [w705 w710]
                                frame False {
                                n495 = Index Array(array=w705, index=1) -> (element=w707:string)
                                n496 = call "PumpStop.vi"("Pump Address"=w707, "Pump COMM Port"=w706) -> ()  [unwired: 9 in, 1 out]
                                }
                                frame True {
                                n497 = Index Array(array=w710, index=1) -> (element=w708:string)
                                n498 = call "PumpDispense.vi"("Flowrate(ul/min)"=w711, "Pump Address"=w708, "Pump COMM Port"=w712) -> ()  [unwired: 7 in, 2 out]
                                }
                                }
                                }
                                frame True {
                                n499 = case shown="True" w715 {
                                tunnel: w714 -> [_ w717]
                                tunnel: w713 -> [w716 w718]
                                frame False {
                                n500 = call <instrlib>:"Stop Pump.vi"("VISA resource name"=w716) -> ()  [unwired: 9 in, 2 out]
                                }
                                frame True {
                                w719 = u16 0 items=["Infuse", "Withdraw"] ("Run Direction (0:Infuse)")
                                w720 = u32 4 items=["milliliters per hour (ml/hr)", "milliliters per minute (ml/min)", "milliliters per second (ml/sec)", "microliters per hour (ul/hr)", "microliters per minute (ul/min)", "microliters per second (ul/sec)", "nanoliters per hour (nl/hr)", "nanoliters per minute (nl/min)", "nanoliters per second (nl/sec)", "picoliters per hour (pl/hr)", "picoliters per minute (pl/min)", "picoliters per second (pl/sec)"] ("Flow Rate Units (1:ml/min)")
                                w721 = u16 0 items=["Infuse", "Withdraw"] ("Pump Direction (0:Infuse)")
                                n501 = call <instrlib>:"Configure Flow Rate & Direction.vi"("VISA resource name"=w718, "Pump Direction (0:Infuse)"=w721, "Flow Rate (5.00)"=w717, "Flow Rate Units (1:ml/min)"=w720) -> ("VISA resource name out"=w722:refnum<visa-resource-name>)  [unwired: 10 in, 1 out]
                                n502 = call <instrlib>:"Start Pump.vi"("Run Direction (0:Infuse)"=w719, "VISA resource name"=w722) -> ()  [unwired: 8 in, 2 out]
                                }
                                }
                                }
                                }
                                n503 = case shown="True" w691 {
                                tunnel: w699 -> [w729 w733]
                                tunnel: w694 -> [_ w734]
                                tunnel: w678 -> [w728 w731]
                                frame False {
                                n504 = Index Array(array=w728, index=0) -> (element=w726:string)
                                n505 = call "PumpStop.vi"("Pump Address"=w726, "Pump COMM Port"=w729) -> ()  [unwired: 9 in, 1 out]
                                }
                                frame True {
                                n506 = Index Array(array=w731, index=0) -> (element=w732:string)
                                n507 = call "PumpDispense.vi"("Flowrate(ul/min)"=w734, "Pump Address"=w732, "Pump COMM Port"=w733) -> ()  [unwired: 7 in, 2 out]
                                }
                                }
                                n508 = case shown="True" w674 {
                                tunnel: w673 -> [_ w725]
                                frame False {
                                n509 = local write "Temperature Control 1"(FALSE) -> ()
                                }
                                frame True {
                                n510 = local write "Temperature SP 1"(w725) -> ()
                                n511 = local write "Temperature Control 1"(TRUE ("Temperature Control 1")) -> ()
                                }
                                }
                              }
                              frame #1 {
                                # "Bay 2"
                                n512 = local read "BAY 2"() -> (w744:u16)
                                n513 = Index Array(array=w753, index=2) -> (element=w751:dbl)
                                n514 = Index Array(array=w753, index=7) -> (element=w738:dbl)
                                n515 = script code="MATLAB script"("T2_SP"=w738) -> ()  [unwired: 1 in, 1 out]
                                n516 = Greater Than 0?(x=w751) -> (x > 0?=w750:bool)
                                n517 = And(x=w750, y=w748) -> (x .and. y?=w749:bool)
                                n518 = Greater Or Equal?(x=w744, y=u16 1) -> (x >= y?=w742:bool)
                                n519 = Less Or Equal?(x=w744, y=u16 4) -> (x <= y?=w747:bool)
                                n520 = And(x=w742, y=w747) -> (x .and. y?=w746:bool)
                                n521 = And(x=w746, y=w748) -> (x .and. y?=w736:bool)
                                n522 = Not Equal?(x=w738, y=23.0) -> (x != y?=w737:bool)
                                n523 = And(x=w736, y=w737) -> (x .and. y?=w735:bool)
                                n524 = case shown="True" w735 {
                                tunnel: w738 -> [_ w766]
                                frame False {
                                n525 = local write "Temperature Control 2"(FALSE) -> ()
                                }
                                frame True {
                                n526 = local write "Temperature Control 2"(TRUE ("Temperature Control 2")) -> ()
                                n527 = local write "Temperature SP 2"(w766) -> ()
                                }
                                }
                                n528 = case shown="True" w749 {
                                tunnel: w751 -> [_ w763]
                                tunnel: w755 -> [w759 w764]
                                tunnel: w740 -> [w756 w761]
                                frame False {
                                n529 = Index Array(array=w756, index=2) -> (element=w757:string)
                                n530 = call "PumpStop.vi"("Pump Address"=w757, "Pump COMM Port"=w759) -> ()  [unwired: 9 in, 1 out]
                                }
                                frame True {
                                n531 = Index Array(array=w761, index=2) -> (element=w760:string)
                                n532 = call "PumpDispense.vi"("Flowrate(ul/min)"=w763, "Pump Address"=w760, "Pump COMM Port"=w764) -> ()  [unwired: 7 in, 2 out]
                                }
                                }
                                n533 = Wait (ms)(milliseconds to wait=u32 300) -> ()  [unwired: 1 out]
                              }
                              frame #2 {
                                # "Bay 3"
                                n534 = local read "BAY 3"() -> (w776:u16)
                                n535 = Index Array(array=w786, index=3) -> (element=w784:dbl)
                                n536 = Not Equal To 0?(x=w784) -> (x != 0?=w783:bool)
                                n537 = Index Array(array=w786, index=8) -> (element=w771:dbl)
                                n538 = script code="MATLAB script"("T3_SP"=w771) -> ()  [unwired: 1 in, 1 out]
                                n539 = Less Or Equal?(x=w776, y=u16 4) -> (x <= y?=w780:bool)
                                n540 = Greater Or Equal?(x=w776, y=u16 1) -> (x >= y?=w777:bool)
                                n541 = And(x=w777, y=w780) -> (x .and. y?=w775:bool)
                                n542 = And(x=w775, y=w781) -> (x .and. y?=w773:bool)
                                n543 = And(x=w783, y=w781) -> (x .and. y?=w782:bool)
                                n544 = Not Equal?(x=w771, y=23.0) -> (x != y?=w772:bool)
                                n545 = And(x=w773, y=w772) -> (x .and. y?=w769:bool)
                                n546 = case shown="False" w782 {
                                tunnel: w784 -> [_ w796]
                                tunnel: w788 -> [w792 w797]
                                tunnel: w768 -> [w789 w793]
                                frame False {
                                n547 = Index Array(array=w789, index=3) -> (element=w790:string)
                                n548 = call "PumpStop.vi"("Pump Address"=w790, "Pump COMM Port"=w792) -> ()  [unwired: 9 in, 1 out]
                                }
                                frame True {
                                n549 = Index Array(array=w793, index=3) -> (element=w794:string)
                                n550 = call "PumpDispense.vi"("Flowrate(ul/min)"=w796, "Pump Address"=w794, "Pump COMM Port"=w797) -> ()  [unwired: 7 in, 2 out]
                                }
                                }
                                n551 = case shown="True" w769 {
                                tunnel: w771 -> [_ w799]
                                frame False {
                                n552 = local write "Temperature Control 3"(FALSE) -> ()
                                }
                                frame True {
                                n553 = local write "Temperature Control 3"(TRUE ("Temperature Control 3")) -> ()
                                n554 = local write "Temperature SP 3"(w799) -> ()
                                }
                                }
                                n555 = Wait (ms)(milliseconds to wait=u32 300) -> ()  [unwired: 1 out]
                              }
                              frame #3 {
                                # "Bay 4"
                                n556 = Index Array(array=w819, index=9) -> (element=w804:dbl)
                                n557 = script code="MATLAB script"("T4_SP"=w804) -> ()  [unwired: 1 in, 1 out]
                                n558 = Index Array(array=w819, index=4) -> (element=w817:dbl)
                                n559 = Not Equal To 0?(x=w817) -> (x != 0?=w816:bool)
                                n560 = local read "BAY 4"() -> (w808:u16)
                                n561 = And(x=w816, y=w814) -> (x .and. y?=w815:bool)
                                n562 = Less Or Equal?(x=w808, y=u16 4) -> (x <= y?=w813:bool)
                                n563 = Greater Or Equal?(x=w808, y=u16 1) -> (x >= y?=w810:bool)
                                n564 = And(x=w810, y=w813) -> (x .and. y?=w809:bool)
                                n565 = And(x=w809, y=w814) -> (x .and. y?=w802:bool)
                                n566 = Not Equal?(x=w804, y=23.0) -> (x != y?=w803:bool)
                                n567 = And(x=w802, y=w803) -> (x .and. y?=w801:bool)
                                n568 = case shown="True" w801 {
                                tunnel: w804 -> [_ w832]
                                frame False {
                                n569 = local write "Temperature Control 4"(FALSE ("Temperature Control 4")) -> ()
                                }
                                frame True {
                                n570 = local write "Temperature SP 4"(w832) -> ()
                                n571 = local write "Temperature Control 4"(TRUE ("Temperature Control 5")) -> ()
                                }
                                }
                                n572 = case shown="True" w815 {
                                tunnel: w821 -> [w825 w830]
                                tunnel: w817 -> [_ w829]
                                tunnel: w806 -> [w822 w826]
                                frame False {
                                n573 = Index Array(array=w822, index=4) -> (element=w823:string)
                                n574 = call "PumpStop.vi"("Pump Address"=w823, "Pump COMM Port"=w825) -> ()  [unwired: 9 in, 1 out]
                                }
                                frame True {
                                n575 = Index Array(array=w826, index=4) -> (element=w827:string)
                                n576 = call "PumpDispense.vi"("Flowrate(ul/min)"=w829, "Pump Address"=w827, "Pump COMM Port"=w830) -> ()  [unwired: 7 in, 2 out]
                                }
                                }
                                n577 = Wait (ms)(milliseconds to wait=u32 300) -> ()  [unwired: 1 out]
                              }
                              frame #4 {
                                # "Bay 5"
                                n578 = Index Array(array=w851, index=5) -> (element=w850:dbl)
                                n579 = Index Array(array=w851, index=4) -> (element=w836:dbl)
                                n580 = script code="MATLAB script"("T5_SP"=w836) -> ()  [unwired: 1 in, 1 out]
                                n581 = local read "BAY 5"() -> (w842:u16)
                                n582 = Not Equal To 0?(x=w850) -> (x != 0?=w849:bool)
                                n583 = And(x=w849, y=w847) -> (x .and. y?=w848:bool)
                                n584 = Less Or Equal?(x=w842, y=u16 4) -> (x <= y?=w846:bool)
                                n585 = Greater Or Equal?(x=w842, y=u16 1) -> (x >= y?=w843:bool)
                                n586 = And(x=w843, y=w846) -> (x .and. y?=w841:bool)
                                n587 = And(x=w841, y=w847) -> (x .and. y?=w835:bool)
                                n588 = Not Equal?(x=w836, y=23.0) -> (x != y?=w837:bool)
                                n589 = And(x=w835, y=w837) -> (x .and. y?=w834:bool)
                                n590 = case shown="True" w834 {
                                tunnel: w836 -> [_ w865]
                                frame False {
                                n591 = local write "Temperature Control 5"(FALSE ("Temperature Control 5")) -> ()
                                }
                                frame True {
                                n592 = local write "Temperature SP 5"(w865) -> ()
                                n593 = local write "Temperature Control 5"(TRUE ("Temperature Control 5")) -> ()
                                }
                                }
                                n594 = case shown="False" w848 {
                                tunnel: w854 -> [w858 w863]
                                tunnel: w850 -> [_ w862]
                                tunnel: w839 -> [w855 w859]
                                frame False {
                                n595 = Index Array(array=w855, index=5) -> (element=w856:string)
                                n596 = call "PumpStop.vi"("Pump Address"=w856, "Pump COMM Port"=w858) -> ()  [unwired: 9 in, 1 out]
                                }
                                frame True {
                                n597 = Index Array(array=w859, index=5) -> (element=w860:string)
                                n598 = call "PumpDispense.vi"("Flowrate(ul/min)"=w862, "Pump Address"=w860, "Pump COMM Port"=w863) -> ()  [unwired: 7 in, 2 out]
                                }
                                }
                                n599 = Wait (ms)(milliseconds to wait=u32 300) -> ()  [unwired: 1 out]
                              }
                            }
                          }
                          frame #1 {
                            # "Wait till Steady State temperature readings on all bays"
                            n600 = while {
                              tunnel: w868 -> [w869]
                              stop <- w870 stop-if-true
                              n601 = flat-sequence {
                                tunnel: [w874] -> w870
                                tunnel: w869 -> [w873]
                                frame #0 {
                                n602 = Wait (ms)(milliseconds to wait=u32 1500) -> ()  [unwired: 1 out]
                                }
                                frame #1 {
                                n603 = local read "Temp SS? 3"() -> (w877:bool)
                                n604 = local read "Temp SS? 4"() -> (w878:bool)
                                n605 = local read "Temp SS? 5"() -> (w879:bool)
                                n606 = local read "Temp SS? 1"() -> (w876:bool)
                                n607 = local read "Temp SS? 2"() -> (w872:bool)
                                n608 = Not(x=w873) -> (.not. x?=w885:bool)
                                n609 = local read "Stop"() -> (w875:bool)
                                n610 = And(x=w877, y=w878) -> (x .and. y?=w881:bool)
                                n611 = And(x=w876, y=w872) -> (x .and. y?=w882:bool)
                                n612 = And(x=w882, y=w881) -> (x .and. y?=w880:bool)
                                n613 = And(x=w880, y=w879) -> (x .and. y?=w883:bool)
                                n614 = Or(x=w885, y=w883) -> (x .or. y?=w884:bool)
                                n615 = Or(x=w884, y=w875) -> (x .or. y?=w874:bool)
                                }
                              }
                            }
                            n616 = local write "Calculate condition"(TRUE ("Calculate condition")) -> ()
                          }
                          frame #2 {
                            n617 = flat-sequence {
                              tunnel: w888 -> [w890]
                              tunnel: [w890] -> w887
                              tunnel: w887 -> [w897]
                              tunnel: [w897] -> w886
                              frame #0 {
                                n618 = local write "Equlibrating Temperature"(TRUE) -> ()
                              }
                              frame #1 {
                                # "Wait 2.5 system volumes"
                                n619 = local read "Number of System Flushes per condtion"() -> (w894:dbl)
                                n620 = local read "Extra system dead volume"() -> (w895:dbl)
                                n621 = script code="start = tic;\nP_tot = P1+P2+P3+P4+P5+P6;\nif P_tot >0\n  extra_res = extr_sys_dead_vol/P_tot;\nelse\n   extra_res =0;\nend\ntotal_sys_res = tau1 + tau2 + tau3 + tau4 + tau5 + extra_res;\ntotal_wait_time = total_sys_res*num_flush_per_cond*60;"("extr_sys_dead_vol"=w895, "num_flush_per_cond"=w894) -> ("??"=w898:errorcluster, "total_wait_time"=w892:dbl, "total_sys_res"=→"Total System Resisdence Time(min)":dbl)  [unwired: 1 in]
                                n622 = Divide(x=w892, y=60.0) -> (x/y=→"total_flush_time":dbl)
                                n623 = while {
                                tunnel: w897 -> [w900]
                                tunnel: w898 -> [w903]
                                stop <- w904 stop-if-true
                                # "Check if system is flushed every 5 seconds"
                                n624 = script code="end1 = toc(start);\nflush_time = 0;\nif end1 > total_wait_time\n   flush_time = 1;\nend\ncurr_wait_time = end1 /60;"("??"=w903) -> ("flush_time"=w907:dbl, "curr_wait_time"=w902:dbl)  [unwired: 1 out]
                                "curr_wait_time" <- w902
                                n625 = Not Equal To 0?(x=w907) -> (x != 0?=w906:bool)
                                n626 = Multiply(x=60.0, y=w902) -> ()  [unwired: 1 out]
                                n627 = local read "Stop"() -> (w909:bool)
                                n628 = Or(x=w906, y=w909) -> (x .or. y?=w905:bool)
                                n629 = Not(x=w900) -> (.not. x?=w899:bool)
                                n630 = Wait (ms)(milliseconds to wait=u32 5000) -> ()  [unwired: 1 out]
                                n631 = Or(x=w905, y=w899) -> (x .or. y?=w904:bool)
                                }
                              }
                            }
                          }
                          frame #3 {
                            # "Collect HPLC Data"
                            n632 = flat-sequence {
                              tunnel: w912 -> [w921]
                              tunnel: w911 -> [w920]
                              tunnel: w910 -> [w919]
                              tunnel: w910 -> [w918]
                              frame #0 {
                                n633 = case shown="True" TRUE {
                                frame False {
                                }
                                frame True {
                                n634 = One Button Dialog(message="Press OK to Analyze Data", button name ("OK")="OK" ("Left Button Text (\"Yes\")")) -> ()  [unwired: 1 out]
                                }
                                }
                                n635 = local write "Flushing System"(TRUE ("Flushing System")) -> ()
                                "System Flushed?" <- TRUE ("System Flushed?")
                              }
                              frame #1 {
                                n636 = flat-sequence {
                                tunnel: w921 -> [w926]
                                tunnel: w920 -> [_]
                                tunnel: w919 -> [w925]
                                tunnel: w918 -> [w924]
                                frame #0 {
                                }
                                frame #1 {
                                n637 = flat-sequence {
                                tunnel: w926 -> [w927]
                                tunnel: w925 -> [w999]
                                tunnel: w926 -> [_]
                                tunnel: [w1020] -> w923
                                tunnel: [w1019] -> w922
                                tunnel: w924 -> [w1018]
                                tunnel: w923 -> [w1053]
                                tunnel: w922 -> [w1052]
                                frame #0 {
                                n638 = local read "COMM Port :: Milligat Pumps"() -> (w929:refnum<visa-resource-name>)
                                n639 = stacked-sequence {
                                tunnel: w929 -> [w932 w944 w962 w967 w976 w989]
                                tunnel: w927 -> [w931 w940 w959 w969 w978 w985]
                                tunnel: 1.0 ("Flowrate(ul/min)") -> [w930 w939 w957 w966 w975 w984]
                                frame #0 {
                                n640 = Index Array(array=w931, index=0) -> (element=w934:dbl)
                                n641 = Greater Than 0?(x=w934) -> (x > 0?=w933:bool)
                                n642 = case shown="True" w933 {
                                tunnel: w932 -> [_ w937]
                                tunnel: w930 -> [_ w936]
                                frame False {
                                }
                                frame True {
                                n643 = call "PumpDispense.vi"("Flowrate(ul/min)"=w936, "Pump Address"="g", "Pump COMM Port"=w937) -> ()  [unwired: 7 in, 2 out]
                                }
                                }
                                }
                                frame #1 {
                                n644 = Index Array(array=w940, index=1) -> (element=w942:dbl)
                                n645 = Greater Than 0?(x=w942) -> (x > 0?=w941:bool)
                                n646 = case shown="True" w941 {
                                tunnel: w939 -> [_ w946]
                                tunnel: w944 -> [_ w945]
                                frame False {
                                }
                                frame True {
                                n647 = local read "Syringe_pump?"() -> (w947:bool)
                                n648 = case shown="True" w947 {
                                tunnel: w946 -> [w948 _]
                                tunnel: w945 -> [w949 _]
                                frame False {
                                n649 = call "PumpDispense.vi"("Flowrate(ul/min)"=w948, "Pump Address"="j", "Pump COMM Port"=w949) -> ()  [unwired: 7 in, 2 out]
                                }
                                frame True {
                                w956 = u16 0 items=["Infuse", "Withdraw"] ("Run Direction (0:Infuse)")
                                w952 = u32 4 items=["milliliters per hour (ml/hr)", "milliliters per minute (ml/min)", "milliliters per second (ml/sec)", "microliters per hour (ul/hr)", "microliters per minute (ul/min)", "microliters per second (ul/sec)", "nanoliters per hour (nl/hr)", "nanoliters per minute (nl/min)", "nanoliters per second (nl/sec)", "picoliters per hour (pl/hr)", "picoliters per minute (pl/min)", "picoliters per second (pl/sec)"] ("Flow Rate Units (1:ml/min)")
                                w953 = u16 0 items=["Infuse", "Withdraw"] ("Pump Direction (0:Infuse)")
                                n650 = local read "COMM Port:: Harvard Syringe Pump"() -> (w954:refnum<visa-resource-name>)
                                n651 = call <instrlib>:"Configure Flow Rate & Direction.vi"("VISA resource name"=w954, "Pump Direction (0:Infuse)"=w953, "Flow Rate (5.00)"=i8 2 ("Pump Address"), "Flow Rate Units (1:ml/min)"=w952) -> ("VISA resource name out"=w955:refnum<visa-resource-name>)  [unwired: 10 in, 1 out]
                                n652 = call <instrlib>:"Start Pump.vi"("Run Direction (0:Infuse)"=w956, "VISA resource name"=w955) -> ()  [unwired: 8 in, 2 out]
                                }
                                }
                                }
                                }
                                }
                                frame #2 {
                                n653 = Index Array(array=w959, index=2) -> (element=w960:dbl)
                                n654 = Greater Than 0?(x=w960) -> (x > 0?=w958:bool)
                                n655 = case shown="True" w958 {
                                tunnel: w962 -> [_ w964]
                                tunnel: w957 -> [_ w963]
                                frame False {
                                }
                                frame True {
                                n656 = call "PumpDispense.vi"("Flowrate(ul/min)"=w963, "Pump Address"="i", "Pump COMM Port"=w964) -> ()  [unwired: 7 in, 2 out]
                                }
                                }
                                }
                                frame #3 {
                                n657 = Index Array(array=w969, index=3) -> (element=w970:dbl)
                                n658 = Greater Than 0?(x=w970) -> (x > 0?=w968:bool)
                                n659 = case shown="True" w968 {
                                tunnel: w967 -> [_ w973]
                                tunnel: w966 -> [_ w972]
                                frame False {
                                }
                                frame True {
                                n660 = call "PumpDispense.vi"("Flowrate(ul/min)"=w972, "Pump Address"="f", "Pump COMM Port"=w973) -> ()  [unwired: 7 in, 2 out]
                                }
                                }
                                }
                                frame #4 {
                                n661 = Index Array(array=w978, index=4) -> (element=w979:dbl)
                                n662 = Greater Than 0?(x=w979) -> (x > 0?=w977:bool)
                                n663 = case shown="True" w977 {
                                tunnel: w976 -> [_ w982]
                                tunnel: w975 -> [_ w981]
                                frame False {
                                }
                                frame True {
                                n664 = call "PumpDispense.vi"("Flowrate(ul/min)"=w981, "Pump Address"="e", "Pump COMM Port"=w982) -> ()  [unwired: 7 in, 2 out]
                                }
                                }
                                }
                                frame #5 {
                                n665 = Index Array(array=w985, index=5) -> (element=w987:dbl)
                                n666 = Greater Than 0?(x=w987) -> (x > 0?=w986:bool)
                                n667 = case shown="True" w986 {
                                tunnel: w989 -> [_ w991]
                                tunnel: w984 -> [_ w990]
                                frame False {
                                }
                                frame True {
                                n668 = call "PumpDispense.vi"("Flowrate(ul/min)"=w990, "Pump Address"="h", "Pump COMM Port"=w991) -> ()  [unwired: 7 in, 2 out]
                                }
                                }
                                }
                                }
                                }
                                frame #1 {
                                n669 = while {
                                stop <- w998 stop-if-true
                                n670 = local read "Phase_Sensor_voltage"() -> (w993:dbl)
                                n671 = script code="organic_phase = 0;\nif start_phase_time \n   start_phase_timer = tic;\n   start_phase_time = 0;\nelse\n  %ignore phase sensor values\n  %if not(phase_sensor_val >2.9 && phase_sensor_val <3.8)\n    %    start_phase_timer = tic;\n   %end\n\n   end_phase_time =  toc(start_phase_timer )\n\n   if end_phase_time > 2\n       organic_phase = 1;\n       start_phase_time = 1;\n   end\n\nend"("phase_sensor_val"=w993) -> ("organic_phase"=w995:dbl)  [unwired: 1 in, 1 out]
                                n672 = local read "Stop"() -> (w997:bool)
                                n673 = Not Equal To 0?(x=w995) -> (x != 0?=w996:bool)
                                n674 = Or(x=w996, y=w997) -> (x .or. y?=w998:bool)
                                n675 = Wait (ms)(milliseconds to wait=u32 300) -> ()  [unwired: 1 out]
                                }
                                }
                                frame #2 {
                                n676 = local read "Stop"() -> (w1001:bool)
                                n677 = Not(x=w1001) -> (.not. x?=w1000:bool)
                                n678 = local read "Sample Valve COMM::Port"() -> (w1002:refnum<visa-resource-name>)
                                n679 = case shown="True" w1000 {
                                tunnel: w1002 -> [_ w1004]
                                tunnel: w999 -> [_ w1003]
                                frame False {
                                }
                                frame True {
                                n680 = flat-sequence {
                                tunnel: w1003 -> [w1005]
                                tunnel: w1004 -> [w1016]
                                frame #0 {
                                n681 = disable-structure shown="Disabled" {
                                frame Disabled {
                                n682 = local read "Sample Valve COMM::Port"() -> (w1012:refnum<visa-resource-name>)
                                n683 = call "NanoValve Inject.vi"("VISA resource name"=w1012) -> ()  [unwired: 10 in, 1 out]
                                }
                                frame Enabled {
                                }
                                }
                                n684 = flat-sequence {
                                tunnel: w1007 -> [w1013]
                                tunnel: [w1013] -> w1006
                                frame #0 {
                                n685 = Wait (ms)(milliseconds to wait=u32 500) -> ()  [unwired: 1 out]
                                }
                                }
                                n686 = call-poly <vilib>:"Digital Write.vi"("Output Value"=FALSE, "DO Channel"=u8 22, "LINX Resource"=w1006) -> ()  [unwired: 7 in, 2 out]
                                n687 = call-poly <vilib>:"Digital Write.vi"("Output Value"=TRUE, "DO Channel"=u8 22, "LINX Resource"=w1005) -> ("LINX Resource"=w1007:T10)  [unwired: 7 in, 1 out]
                                }
                                frame #1 {
                                n688 = Wait (ms)(milliseconds to wait=u32 2000) -> ()  [unwired: 1 out]
                                }
                                frame #2 {
                                n689 = disable-structure shown="Disabled" {
                                disable-tunnel: w1016 -> [w1017 _]
                                frame Disabled {
                                n690 = call "NanoValve Load.vi"("VISA resource name"=w1017) -> ()  [unwired: 10 in, 1 out]
                                }
                                frame Enabled {
                                }
                                }
                                }
                                }
                                }
                                }
                                }
                                frame #3 {
                                n691 = local read "Stop"() -> (w1023:bool)
                                n692 = local read "Bay Parameters"() -> (w1019:T2)
                                n693 = Unbundle By Name(w1019) -> ("Hplc Wait time(min)"=w1021:dbl)
                                n694 = Not(x=w1023) -> (.not. x?=w1022:bool)
                                n695 = case shown="True" w1022 {
                                tunnel: w1021 -> [_ w1028]
                                tunnel: [errorcluster {"status"=FALSE, "code"=0, "source"=""} ("error out") w1027] -> w1020
                                tunnel: w1019 -> [_ w1026]
                                tunnel: w1018 -> [_ w1025]
                                frame False {
                                }
                                frame True {
                                n696 = flat-sequence {
                                tunnel: w1028 -> [w1030]
                                tunnel: w1025 -> [w1045]
                                tunnel: [w1050] -> w1027
                                tunnel: w1026 -> [w1049]
                                frame #0 {
                                # "Wait till for HPLC Method"
                                n697 = script code="start = tic;"() -> ("??"=w1029:errorcluster)  [unwired: 1 in]
                                n698 = while {
                                tunnel: w1030 -> [w1032]
                                tunnel: w1029 -> [w1031]
                                stop <- w1038 stop-if-true
                                n699 = Multiply(x=w1032, y=60.0) -> (x*y=w1033:dbl)
                                n700 = script code="end1 = toc(start);\nflush_time = 0;\nif end1 > hplc_wait_time\n   flush_time = 1;\nend"("??"=w1031, "hplc_wait_time"=w1033) -> ("flush_time"=w1035:dbl)  [unwired: 1 out]
                                n701 = local read "Stop"() -> (w1037:bool)
                                n702 = Not Equal To 0?(x=w1035) -> (x != 0?=w1036:bool)
                                n703 = Or(x=w1036, y=w1037) -> (x .or. y?=w1038:bool)
                                }
                                }
                                frame #1 {
                                n704 = flat-sequence {
                                tunnel: w1040 -> [w1046]
                                tunnel: [w1046] -> w1039
                                frame #0 {
                                n705 = Wait (ms)(milliseconds to wait=u32 500) -> ()  [unwired: 1 out]
                                }
                                }
                                n706 = call-poly <vilib>:"Digital Write.vi"("Output Value"=FALSE, "DO Channel"=u8 24, "LINX Resource"=w1045) -> ("LINX Resource"=w1040:T10)  [unwired: 7 in, 1 out]
                                n707 = call-poly <vilib>:"Digital Write.vi"("Output Value"=TRUE, "DO Channel"=u8 24, "LINX Resource"=w1039) -> ()  [unwired: 7 in, 2 out]
                                }
                                frame #2 {
                                n708 = Wait (ms)(milliseconds to wait=u32 30000) -> ()  [unwired: 1 out]
                                }
                                frame #3 {
                                n709 = Unbundle By Name(w1049) -> ("hplc File Name"=w1051:string)
                                n710 = call "hplc_analyze.vi"("File Path"=w1051) -> ("error out"=w1050:errorcluster)  [unwired: 10 in]
                                }
                                }
                                }
                                }
                                }
                                frame #4 {
                                n711 = Unbundle By Name(w1053) -> ("status"=w1054:bool)
                                n712 = case shown="True" w1054 {
                                tunnel: w1052 -> [_ w1055]
                                frame False {
                                }
                                frame True {
                                n713 = while {
                                tunnel: w1055 -> [w1057]
                                stop <- w1056 stop-if-true
                                w1062 = "An error occured while trying to read HPLC data. " ("message")
                                n714 = local write "Error Message"(w1062) -> ()
                                n715 = call <vilib>:"Three Button Dialog.vi"("Right Button Text (\"Cancel\")"="STOP EXPs" ("F button name (\"Cancel\")"), "Center Button Text (\"No\")"="REDO" ("T button name (\"OK\")"), "Left Button Text (\"Yes\")"="REREAD" ("T button name (\"OK\")"), "message"=w1062) -> ("Which Button?"=w1058:T19)  [unwired: 7 in]
                                n716 = case shown="\"Left Button\"" w1058 {
                                tunnel: w1057 -> [_ _ w1069 _]
                                tunnel: [TRUE TRUE w1068 w1071] -> w1056
                                frame "Right Button" {
                                w1063 = TRUE ("Setup Error")
                                n717 = local write "System Error"(w1063) -> ()
                                n718 = local write "Setup Error"(w1063) -> ()
                                n719 = script code="system_error = 1"() -> ()  [unwired: 1 in, 1 out]
                                n720 = local write "Stop"(w1063) -> ()
                                }
                                frame "Center Button" {
                                n721 = script code="redo = true;\nopt_ctr = 1;\nCurrExp = CurrExp + 1;\nncall0 = ncall0 +1;\nif req_ctr == req_tot\n       opt_ctr = 3;\n  else\n     req_ctr = req_ctr +1;\nend"() -> ()  [unwired: 1 in, 1 out]
                                }
                                frame "Left Button" {
                                n722 = Unbundle By Name(w1069) -> ("hplc File Name"=w1070:string)
                                n723 = call "hplc_analyze.vi"("File Path"=w1070) -> ("error out"=w1066:errorcluster)  [unwired: 10 in]
                                n724 = Unbundle By Name(w1066) -> ("status"=w1067:bool)
                                n725 = Not(x=w1067) -> (.not. x?=w1068:bool)
                                }
                                frame "Window Close" {
                                w1071 = TRUE
                                n726 = local write "Setup Error"(w1071) -> ()
                                n727 = script code="system_error = 1"() -> ()  [unwired: 1 in, 1 out]
                                n728 = local write "Stop"(w1071) -> ()
                                }
                                }
                                }
                                }
                                }
                                }
                                frame #5 {
                                n729 = disable-structure shown="Disabled" {
                                frame Disabled {
                                n730 = flat-sequence {
                                tunnel: w1073 -> [w1078]
                                tunnel: [w1078] -> w1072
                                frame #0 {
                                n731 = Wait (ms)(milliseconds to wait=u32 500) -> ()  [unwired: 1 out]
                                }
                                }
                                n732 = call-poly <vilib>:"Digital Write.vi"("Output Value"=FALSE, "DO Channel"=u8 22) -> ("LINX Resource"=w1073:T10)  [unwired: 8 in, 1 out]
                                n733 = call-poly <vilib>:"Digital Write.vi"("Output Value"=TRUE, "DO Channel"=u8 22, "LINX Resource"=w1072) -> ()  [unwired: 7 in, 2 out]
                                }
                                frame Enabled {
                                }
                                }
                                }
                                }
                                }
                                }
                              }
                              frame #2 {
                                n734 = local read "Stop"() -> (w1081:bool)
                                n735 = local write "HPLC Analysis"(TRUE ("HPLC Analysis")) -> ()
                                n736 = Not(x=w1081) -> (.not. x?=w1080:bool)
                                n737 = case shown="True" w1080 {
                                frame False {
                                }
                                frame True {
                                n738 = script code="C_measured =Conc;\nFvalues(end +1,:) = [Conc];"() -> ()  [unwired: 1 in, 1 out]
                                }
                                }
                              }
                            }
                          }
                          frame #4 {
                            n739 = local read "Stop"() -> (w1084:bool)
                            n740 = Not(x=w1084) -> (.not. x?=w1083:bool)
                            n741 = case shown="True" w1083 {
                              tunnel: [1.0 w1095] -> w1085
                              frame False {
                              }
                              frame True {
                                # "Save data to excel file"
                                n742 = local read "Bay Parameters"() -> (w1093:T2)
                                n743 = Unbundle By Name(w1093) -> ("Total Number of Experiments 2"=w1092:dbl)
                                n744 = script code="analyze_labview_results"("ncall"=w1092) -> ("terminate"=w1095:dbl, "ncall0"=w1094:dbl, "experiment_history"=w1090:dbl[][], "Pbest"=w1088:dbl[], "Tbest"=w1089:dbl[], "best_exp_num"=w1087:dbl)  [unwired: 1 in, 1 out]
                                n745 = local write "Flowrates(ul/min)_best"(w1088) -> ()
                                n746 = local write "temperature_best"(w1089) -> ()
                                n747 = local write "best_exp_num"(w1087) -> ()
                                n748 = local write "Current Experiment"(w1094) -> ()
                                n749 = local write "Total Number of Experiments"(w1092) -> ()
                                n750 = call-poly <vilib>:"Array To Matrix.vi"("Real 2D Array"=w1090) -> ("Real Matrix"=w1091:T18)
                                n751 = local write "experiment history"(w1091) -> ()
                              }
                            }
                          }
                          frame #5 {
                            n752 = local read "Num_exp_till_pause"() -> (w1097:i32)
                            n753 = Increment(x=w1097) -> (x+1=w1096:i32)
                            n754 = local write "Num_exp_till_pause"(w1096) -> ()
                          }
                          frame #6 {
                            # "Pause System"
                            n755 = local read "Bay Parameters"() -> (w1105:T2)
                            n756 = Unbundle By Name(w1105) -> ("Num_conditons_per_wait"=w1104:dbl)
                            n757 = local read "Num_exp_till_pause"() -> (w1103:i32)
                            n758 = Equal?(x=w1104, y=w1103) -> (x = y?=w1102:bool)
                            n759 = local read "Run_Stop_cluster"() -> (w1099:T7)
                            n760 = Unbundle By Name(w1099) -> ("Stop Run Button"=w1101:bool)
                            n761 = Or(x=w1101, y=w1102) -> (x .or. y?=w1100:bool)
                            n762 = case shown="True" w1100 {
                              tunnel: w1104 -> [w1108 _]
                              tunnel: w1103 -> [w1109 _]
                              tunnel: w1099 -> [_ w1111]
                              frame False {
                                n763 = Greater?(x=w1109, y=w1108) -> (0:w1107:bool)
                                n764 = case shown="True" w1107 {
                                frame False {
                                }
                                frame True {
                                n765 = local write "Num_exp_till_pause"(0 ("Num_exp_till_pause")) -> ()
                                }
                                }
                              }
                              frame True {
                                n766 = flat-sequence {
                                tunnel: w1111 -> [w1139]
                                frame #0 {
                                w1115 = string[] ["e", "f", "g", "h", "i", "j"]
                                # "Turn off pumps and stop controling temperature"
                                n767 = stacked-sequence {
                                frame #0 {
                                n768 = local write "Temperature Control 1"(FALSE ("Temperature Control 1")) -> ()
                                }
                                frame #1 {
                                n769 = local write "Temperature Control 2"(FALSE ("Temperature Control 2")) -> ()
                                }
                                frame #2 {
                                n770 = local write "Temperature Control 3"(FALSE ("Temperature Control 3")) -> ()
                                }
                                frame #3 {
                                n771 = local write "Temperature Control 4"(FALSE ("Temperature Control 4")) -> ()
                                }
                                frame #4 {
                                n772 = local write "Temperature Control 5"(FALSE ("Temperature Control 5")) -> ()
                                }
                                }
                                n773 = local read "COMM Port:: Harvard Syringe Pump"() -> (w1113:refnum<visa-resource-name>)
                                n774 = local read "Syringe_pump?"() -> (w1112:bool)
                                n775 = local read "COMM Port :: Milligat Pumps"() -> (w1114:refnum<visa-resource-name>)
                                n776 = Array Size(array=w1115) -> (size(s)=w1116:i32)
                                n777 = case shown="True" w1112 {
                                tunnel: w1113 -> [_ w1124]
                                frame False {
                                }
                                frame True {
                                n778 = call <instrlib>:"Stop Pump.vi"("VISA resource name"=w1124) -> ()  [unwired: 9 in, 2 out]
                                }
                                }
                                n779 = for {
                                N: w1116 -> [_]
                                tunnel: w1115 -> [w1122] mode=indexing
                                tunnel: w1114 -> [w1123]
                                n780 = call "PumpStop.vi"("Pump Address"=w1122, "Pump COMM Port"=w1123) -> ()  [unwired: 9 in, 1 out]
                                }
                                }
                                frame #1 {
                                n781 = local read "Stop"() -> (w1127:bool)
                                n782 = Not(x=w1127) -> (.not. x?=w1126:bool)
                                n783 = case shown="True" w1126 {
                                frame False {
                                }
                                frame True {
                                n784 = while {
                                stop <- w1133 stop-if-true
                                # "Wait till user confirms system resume"
                                n785 = Two Button Dialog(message="System is currently paused. Refill Syringes, flush lines, then press OK to continue optimization.\nOr Redo to repeat condition ", 1:"REDO" ("F button name (\"Cancel\")"), 2:"OK" ("Left Button Text (\"Yes\")")) -> (T button?=w1129:bool)
                                n786 = case shown="False" w1129 {
                                tunnel: [TRUE TRUE] -> w1128
                                frame False {
                                n787 = script code="redo = true;"() -> ()  [unwired: 1 in, 1 out]
                                }
                                frame True {
                                }
                                }
                                n788 = local read "Stop"() -> (w1134:bool)
                                n789 = Or(x=w1128, y=w1134) -> (x .or. y?=w1133:bool)
                                }
                                }
                                }
                                n790 = local write "stop_xl_write"(TRUE ("stop_xl_write")) -> ()
                                }
                                frame #2 {
                                n791 = local write "Num_exp_till_pause"(0 ("Num_exp_till_pause")) -> ()
                                n792 = Bundle By Name(cluster=w1139, "Stop Run Button"=FALSE) -> (w1137:T7)
                                n793 = local write "Run_Stop_cluster"(w1137) -> ()
                                }
                                }
                              }
                            }
                          }
                          frame #7 {
                            w1142 = FALSE
                            n794 = local write "Equlibrating Temperature"(w1142) -> ()
                            n795 = local write "Calculate condition"(w1142) -> ()
                            n796 = local write "Flushing System"(w1142) -> ()
                            n797 = local write "HPLC Analysis"(w1142) -> ()
                            n798 = local write "stop_xl_write"(TRUE ("stop_xl_write")) -> ()
                          }
                        }
                        n799 = while {
                          stop <- w1169 stop-if-true
                          n800 = flat-sequence {
                            frame #0 {
                              n801 = script code="save_excel_time_data;"() -> ()  [unwired: 1 in, 1 out]
                            }
                            frame #1 {
                              n802 = Wait (ms)(milliseconds to wait=u32 30000) -> ()  [unwired: 1 out]
                            }
                          }
                          n803 = local read "Stop"() -> (w1170:bool)
                          n804 = local read "stop_xl_write"() -> (w1168:bool)
                          n805 = Or(x=w1168, y=w1170) -> (x .or. y?=w1169:bool)
                        }
                      }
                    }
                  }
                }
                n806 = Greater?(x=w609, y=w610) -> (0:w617:bool)
                n807 = Equal?(x=w615, y=1.0) -> (x = y?=w611:bool)
                n808 = local read "Stop"() -> (w618:bool)
                n809 = Or(x=w618, y=w617) -> (x .or. y?=w614:bool)
                n810 = Or(x=w611, y=w614) -> (x .or. y?=w613:bool)
                n811 = case shown="True" w611 {
                  frame False {
                  }
                  frame True {
                    w622 = u16 2 items=["System  Error", "System Running", "System Standby"] ("System Status")
                    n812 = local write "Stop"(TRUE ("Stop")) -> ()
                    n813 = local write "System Status"(w622) -> ()
                  }
                }
                "Optimization_loop_index" <- w619
              }
            }
          }
          n814 = while {
            tunnel: w597 -> [w1265]
            stop <- w1268 stop-if-true
            n815 = local read "Temperature Control 3"() -> (w1266:bool)
            n816 = local read "running?"() -> (w1264:bool)
            n817 = And(x=w1264, y=w1266) -> (x .and. y?=w1267:bool)
            n818 = case shown="False" w1267 {
              tunnel: w1265 -> [_ w1271]
              frame False {
                n819 = local write "Temp SS? 3"(TRUE) -> ()
              }
              frame True {
                # "Bay 3 Temperature Controller"
                n820 = local read "Temperature SP 3"() -> (w1272:dbl)
                n821 = local read "Temperature 3"() -> (w1275:dbl)
                n822 = Subtract(x=w1275, y=w1272) -> (x-y=w1284:dbl)
                n823 = Absolute Value(x=w1284) -> (abs(x)=w1286:dbl)
                n824 = Less Or Equal?(x=w1286, y=1.2) -> (x <= y?=w1283:bool)
                n825 = local write "Temp SS? 3"(w1283) -> ()
                n826 = local read "SSR Duration 3"() -> (w1293:dbl)
                n827 = call-poly <vilib>:"PID Online Autotuning.vi"("setpoint"=w1272, "manipulated variable"=w1293, "autotuning parameters"=T9 {"type of controller"=enum."PID", "relay cycles"=3, "relay amplitude"=1.0, "control specifications"=enum."Normal", "PV noise level"=0.1} ("Autotuning Parameters R1"), "process variable"=w1275, "PID gains in"=T8 {"Proportional gain Kc"=0.38538, "Integral time Ti (sec)"=0.524375, "Derivative time Ti (sec)"=0.12585} ("PID gains 2")) -> ("setpoint out"=w1291:dbl, "process variable out"=w1292:dbl, "PID gains out"=w1295:T17)  [unwired: 6 in, 2 out]
                n828 = Greater?(x=w1272, y=w1275) -> (0:w1282:bool)
                n829 = call <vilib>:"PID Autotuning (Temperature).vi"("desired temperature"=w1291, "measured temperature"=w1292, "PID gains in"=w1295, "output range"=cluster{"output high":dbl, "output low":dbl} {"output high"=3.0, "output low"=-1.0} ("Output range")) -> ("output"=w1288:dbl)  [unwired: 12 in, 3 out]
                n830 = Multiply(x=1000.0, y=w1288) -> (x*y=w1290:dbl)
                n831 = local write "SSR Duration 3"(w1288) -> ()
                n832 = Greater Than 0?(x=w1290) -> (x > 0?=w1281:bool)
                n833 = And(x=w1281, y=w1282) -> (x .and. y?=w1279:bool)
                n834 = Subtract(x=w1275, y=10.0) -> (x-y=w1277:dbl)
                n835 = Less?(x=w1277, y=w1272) -> (x < y?=w1280:bool)
                n836 = And(x=w1280, y=w1279) -> (x .and. y?=w1278:bool)
                n837 = case shown="True" w1278 {
                  tunnel: [errorcluster {"status"=FALSE, "code"=0, "source"=""} ("error out") w1307] -> _
                  tunnel: 4 -> [_ w1305]
                  tunnel: w1290 -> [w1301 w1306]
                  tunnel: [0.0 w1309] -> w1273
                  tunnel: w1272 -> [_ w1308]
                  tunnel: w1271 -> [_ w1304]
                  frame False {
                    n838 = Absolute Value(x=w1301) -> (abs(x)=w1302:dbl)
                    n839 = Wait (ms)(milliseconds to wait=w1302) -> ()  [unwired: 1 out]
                  }
                  frame True {
                    n840 = call "TurnOnRelayArduino.vi"("channel"=w1305, "duration"=w1306, "LINX Resource"=w1304) -> ("error out"=w1307:errorcluster)  [unwired: 7 in, 1 out]
                    n841 = script code="tempdiff3= SP3 - T3;\nif tempdiff3 > 10\n  if slope3 < .01\n     temp_check3 = temp_check3 + 1;\n  else\n      temp_check3 =0;\n  end\nend\n\nif temp_check3 > 9\n  temp_error3 = 1\nend"("SP3"=w1308) -> ("temp_error3"=w1309:dbl)  [unwired: 1 in, 1 out]
                  }
                }
                n842 = Not Equal To 0?(x=w1273) -> (x != 0?=w1274:bool)
                n843 = case shown="True" w1274 {
                  frame False {
                  }
                  frame True {
                    n844 = local write "Error Message"("Bay 3 Temperature Heating Error") -> ()
                  }
                }
                n845 = case shown="True" w1274 {
                  tunnel: w1274 -> [_ w1299]
                  frame False {
                  }
                  frame True {
                    n846 = local write "System Error"(w1299) -> ()
                    n847 = local write "Stop"(w1299) -> ()
                  }
                }
              }
            }
            n848 = Wait (ms)(milliseconds to wait=u32 400) -> ()  [unwired: 1 out]
            n849 = local read "Stop"() -> (w1268:bool)
          }
          n850 = while {
            tunnel: w597 -> [w1219]
            stop <- w1222 stop-if-true
            n851 = local read "running?"() -> (w1218:bool)
            n852 = Wait (ms)(milliseconds to wait=u32 400) -> ()  [unwired: 1 out]
            n853 = local read "Temperature Control 4"() -> (w1221:bool)
            n854 = And(x=w1218, y=w1221) -> (x .and. y?=w1220:bool)
            n855 = case shown="False" w1220 {
              tunnel: w1219 -> [_ w1225]
              frame False {
                n856 = local write "Temp SS? 4"(TRUE ("Temp SS? 4")) -> ()
              }
              frame True {
                # "Bay 4 Temperature Controller"
                n857 = local read "Temperature SP 4"() -> (w1228:dbl)
                n858 = local read "Temperature 4"() -> (w1231:dbl)
                n859 = Subtract(x=w1231, y=w1228) -> (x-y=w1238:dbl)
                n860 = Absolute Value(x=w1238) -> (abs(x)=w1240:dbl)
                n861 = Less Or Equal?(x=w1240, y=1.2) -> (x <= y?=w1237:bool)
                n862 = local write "Temp SS? 4"(w1237) -> ()
                n863 = local read "SSR Duration 4"() -> (w1241:dbl)
                n864 = call-poly <vilib>:"PID Online Autotuning.vi"("setpoint"=w1228, "manipulated variable"=w1241, "autotuning parameters"=T9 {"type of controller"=enum."PID", "relay cycles"=3, "relay amplitude"=1.0, "control specifications"=enum."Normal", "PV noise level"=0.1} ("Autotuning Parameters R1"), "process variable"=w1231, "PID gains in"=T8 {"Proportional gain Kc"=0.38538, "Integral time Ti (sec)"=0.524375, "Derivative time Ti (sec)"=0.12585} ("PID gains 2")) -> ("setpoint out"=w1243:dbl, "process variable out"=w1244:dbl, "PID gains out"=w1246:T17)  [unwired: 6 in, 2 out]
                n865 = call <vilib>:"PID Autotuning (Temperature).vi"("desired temperature"=w1243, "measured temperature"=w1244, "PID gains in"=w1246, "output range"=cluster{"output high":dbl, "output low":dbl} {"output high"=3.0, "output low"=-1.0} ("Output range")) -> ("output"=w1242:dbl)  [unwired: 12 in, 3 out]
                n866 = Subtract(x=w1231, y=10.0) -> (x-y=w1230:dbl)
                n867 = Less?(x=w1230, y=w1228) -> (x < y?=w1232:bool)
                n868 = Multiply(x=1000.0, y=w1242) -> (x*y=w1250:dbl)
                n869 = Greater?(x=w1228, y=w1231) -> (0:w1236:bool)
                n870 = Greater Than 0?(x=w1250) -> (x > 0?=w1235:bool)
                n871 = local write "SSR Duration 4"(w1242) -> ()
                n872 = And(x=w1235, y=w1236) -> (x .and. y?=w1234:bool)
                n873 = And(x=w1232, y=w1234) -> (x .and. y?=w1233:bool)
                n874 = case shown="True" w1233 {
                  tunnel: [errorcluster {"status"=FALSE, "code"=0, "source"=""} ("error out") w1261] -> _
                  tunnel: 5 -> [_ w1259]
                  tunnel: w1250 -> [w1255 w1260]
                  tunnel: w1228 -> [_ w1263]
                  tunnel: [0.0 w1262] -> w1227
                  tunnel: w1225 -> [_ w1258]
                  frame False {
                    n875 = Absolute Value(x=w1255) -> (abs(x)=w1256:dbl)
                    n876 = Wait (ms)(milliseconds to wait=w1256) -> ()  [unwired: 1 out]
                  }
                  frame True {
                    n877 = call "TurnOnRelayArduino.vi"("channel"=w1259, "duration"=w1260, "LINX Resource"=w1258) -> ("error out"=w1261:errorcluster)  [unwired: 7 in, 1 out]
                    n878 = script code="tempdiff4= SP4 - T4;\nif tempdiff4 > 10\n  if slope4 < .01\n     temp_check4 = temp_check4 + 1;\n  else\n      temp_check4 =0;\n  end\nend\n\nif temp_check4 > 9\n  temp_error4 = 1\nend"("SP4"=w1263) -> ("temp_error4"=w1262:dbl)  [unwired: 1 in, 1 out]
                  }
                }
                n879 = Not Equal To 0?(x=w1227) -> (x != 0?=w1226:bool)
                n880 = case shown="True" w1226 {
                  frame False {
                  }
                  frame True {
                    n881 = local write "Error Message"("Bay 4 Temperature Heating Error") -> ()
                  }
                }
                n882 = case shown="True" w1226 {
                  tunnel: w1226 -> [_ w1253]
                  frame False {
                  }
                  frame True {
                    n883 = local write "System Error"(w1253) -> ()
                    n884 = local write "Stop"(w1253) -> ()
                  }
                }
              }
            }
            n885 = local read "Stop"() -> (w1222:bool)
          }
          n886 = while {
            stop <- w602 stop-if-true
            n887 = script code="TempArr1=circshift(TempArr1,9);\nTempArr2=circshift(TempArr2,9);\nTempArr3=circshift(TempArr3,9);\nTempArr4=circshift(TempArr4,9);\nTempArr5=circshift(TempArr5,9);\n\nTempArr1(10)=T1;\nTempArr2(10)=T2;\nTempArr3(10)=T3;\nTempArr4(10)=T4;\nTempArr5(10)=T5;\n\n[slope1 temp] = polyfit([1,2,3,4,5,6,7,8,9,10]',TempArr1,1);\nslope1 = slope1(1);\n[slope2 temp] = polyfit([1,2,3,4,5,6,7,8,9,10]',TempArr2,1);\nslope2= slope2(1);\n[slope3 temp] = polyfit([1,2,3,4,5,6,7,8,9,10]',TempArr3,1);\nslope3 = slope3(1);\n[slope4 temp] = polyfit([1,2,3,4,5,6,7,8,9,10]',TempArr4,1);\nslope4 = slope4(1);\n[slope5 temp] = polyfit([1,2,3,4,5,6,7,8,9,10]',TempArr5,1);\nslope5 = slope5(1);"() -> ()  [unwired: 1 in, 1 out]
            n888 = Wait (ms)(milliseconds to wait=u32 600) -> ()  [unwired: 1 out]
            n889 = local read "Stop"() -> (w602:bool)
          }
          n890 = while {
            tunnel: w597 -> [w1173]
            stop <- w1176 stop-if-true
            n891 = local read "running?"() -> (w1172:bool)
            n892 = local read "Temperature Control 5"() -> (w1174:bool)
            n893 = And(x=w1172, y=w1174) -> (x .and. y?=w1175:bool)
            n894 = case shown="True" w1175 {
              tunnel: w1173 -> [_ w1179]
              frame False {
                n895 = local write "Temp SS? 5"(TRUE ("Temp SS? 5")) -> ()
              }
              frame True {
                # "Bay 5 Temperature Controller"
                n896 = local read "SSR Duration 5"() -> (w1195:dbl)
                n897 = local read "Temperature SP 5"() -> (w1181:dbl)
                n898 = local read "Temperature 5"() -> (w1184:dbl)
                n899 = Subtract(x=w1184, y=w1181) -> (x-y=w1192:dbl)
                n900 = Absolute Value(x=w1192) -> (abs(x)=w1194:dbl)
                n901 = Less Or Equal?(x=w1194, y=1.2) -> (x <= y?=w1191:bool)
                n902 = local write "Temp SS? 5"(w1191) -> ()
                n903 = call-poly <vilib>:"PID Online Autotuning.vi"("setpoint"=w1181, "manipulated variable"=w1195, "autotuning parameters"=T9 {"type of controller"=enum."PID", "relay cycles"=3, "relay amplitude"=1.0, "control specifications"=enum."Normal", "PV noise level"=0.1} ("Autotuning Parameters R1"), "process variable"=w1184, "PID gains in"=T8 {"Proportional gain Kc"=0.38538, "Integral time Ti (sec)"=0.524375, "Derivative time Ti (sec)"=0.12585} ("PID gains 2")) -> ("setpoint out"=w1197:dbl, "process variable out"=w1198:dbl, "PID gains out"=w1200:T17)  [unwired: 6 in, 2 out]
                n904 = call <vilib>:"PID Autotuning (Temperature).vi"("desired temperature"=w1197, "measured temperature"=w1198, "PID gains in"=w1200, "output range"=cluster{"output high":dbl, "output low":dbl} {"output high"=3.0, "output low"=-1.0} ("Output range")) -> ("output"=w1196:dbl)  [unwired: 12 in, 3 out]
                n905 = Multiply(x=1000.0, y=w1196) -> (x*y=w1204:dbl)
                n906 = Greater?(x=w1181, y=w1184) -> (0:w1189:bool)
                n907 = Greater Than 0?(x=w1204) -> (x > 0?=w1190:bool)
                n908 = local write "SSR Duration 5"(w1196) -> ()
                n909 = And(x=w1190, y=w1189) -> (x .and. y?=w1187:bool)
                n910 = Subtract(x=w1184, y=10.0) -> (x-y=w1185:dbl)
                n911 = Greater?(x=w1185, y=w1181) -> (0:w1188:bool)
                n912 = And(x=w1188, y=w1187) -> (x .and. y?=w1186:bool)
                n913 = case shown="True" w1186 {
                  tunnel: [errorcluster {"status"=FALSE, "code"=0, "source"=""} ("error out") w1215] -> _
                  tunnel: 6 -> [_ w1212]
                  tunnel: w1204 -> [w1209 w1213]
                  tunnel: [0.0 w1217] -> w1182
                  tunnel: w1181 -> [_ w1216]
                  tunnel: w1179 -> [_ w1214]
                  frame False {
                    n914 = Absolute Value(x=w1209) -> (abs(x)=w1210:dbl)
                    n915 = Wait (ms)(milliseconds to wait=w1210) -> ()  [unwired: 1 out]
                  }
                  frame True {
                    n916 = call "TurnOnRelayArduino.vi"("channel"=w1212, "duration"=w1213, "LINX Resource"=w1214) -> ("error out"=w1215:errorcluster)  [unwired: 7 in, 1 out]
                    n917 = script code="tempdiff5= SP5 - T5;\n\nif tempdiff5 > 10\n  if slope5 < .01\n     temp_check5 = temp_check5 + 1;\n  else\n      temp_check5 =0;\n  end\nend\n\nif temp_check5 >9\n  temp_error5 = 1\nend"("SP5"=w1216) -> ("temp_error5"=w1217:dbl)  [unwired: 1 in, 1 out]
                  }
                }
                n918 = Not Equal To 0?(x=w1182) -> (x != 0?=w1180:bool)
                n919 = case shown="True" w1180 {
                  frame False {
                  }
                  frame True {
                    n920 = local write "Error Message"("Bay 5 Temperature Heating Error") -> ()
                  }
                }
                n921 = case shown="True" w1180 {
                  tunnel: w1180 -> [_ w1207]
                  frame False {
                  }
                  frame True {
                    n922 = local write "Stop"(w1207) -> ()
                    n923 = local write "System Error"(w1207) -> ()
                  }
                }
              }
            }
            n924 = Wait (ms)(milliseconds to wait=u32 400) -> ()  [unwired: 1 out]
            n925 = local read "Stop"() -> (w1176:bool)
          }
        }
      }
      n926 = local read "IR Sensor Device"() -> (w62:T6)
      n927 = while {
        tunnel: errorcluster {"status"=FALSE, "code"=0, "source"=""} ("error out") -> [w140]
        tunnel: w62 -> [w159]
        stop <- w180 stop-if-true
        w137 = u8 7 items=["RAM IR raw  Ch1"=4, "RAM IR raw  Ch2"=5, "RAM T_A"=6, "RAM T_OBJ1"=7, "RAM T_OBJ2"=8, "EEPROM_To_max"=32, "EEPROM_To_min"=33, "EEPROM_PWM_CTRL"=34, "EEPROM_Ta_range"=35, "EEPROM_Emissivity_CorrCoeff"=36, "EEPROM_SMBus Address"=46, "EEPROM_ConfigReg"=37] ("Melexis_Cmmds")
        # "Bay 5 Temperature Read"
        # "Bay 4 Temperature Read"
        # "Bay 3 Temperature Read"
        # "Bay 2 Temperature Read"
        # "Bay 1 Temperature Read"
        n928 = local read "Stop"() -> (w180:bool)
        n929 = call "IRSensorNIRead.vi"("error in (no error)"=w140, "Melexis_Cmmds"=w137, "Address"=u8 1, "device reference"=w159) -> ("error out"=w162:errorcluster, "Temperature"=w160:dbl, "device reference out"=w158:T6)  [unwired: 5 in]
        n930 = local write "error out"(w162) -> ()
        n931 = Unbundle By Name(w162) -> ("status"=w161:bool)
        n932 = call-poly <vilib>:"PID Control Input Filter.vi"("input"=w160) -> ("output"=w173:dbl)  [unwired: 4 in]
        n933 = case shown="False" w161 {
          tunnel: w172 -> [w189 _]
          tunnel: [w189 w190] -> w177
          frame False {
            n934 = local write "Temperature 1"(w189) -> ()
          }
          frame True {
            n935 = local read "Temperature 1"() -> (w190:dbl)
          }
        }
        n936 = flat-sequence {
          tunnel: w173 -> [w203]
          tunnel: [w203] -> w172
          tunnel: w158 -> [w202]
          tunnel: [w202] -> w157
          frame #0 {
            n937 = Wait (ms)(milliseconds to wait=u32 100) -> ()  [unwired: 1 out]
          }
        }
        n938 = call "IRSensorNIRead.vi"("error in (no error)"=w140, "Melexis_Cmmds"=w137, "Address"=u8 2, "device reference"=w157) -> ("error out"=w149:errorcluster, "Temperature"=w150:dbl, "device reference out"=w152:T6)  [unwired: 5 in]
        n939 = local write "error out"(w149) -> ()
        n940 = Unbundle By Name(w149) -> ("status"=w154:bool)
        n941 = call-poly <vilib>:"PID Control Input Filter.vi"("input"=w150) -> ("output"=w171:dbl)  [unwired: 4 in]
        n942 = case shown="True" w154 {
          tunnel: w170 -> [w187 _]
          tunnel: [w187 w188] -> w176
          frame False {
            n943 = local write "Temperature 2"(w187) -> ()
          }
          frame True {
            n944 = local read "Temperature 2"() -> (w188:dbl)
          }
        }
        n945 = flat-sequence {
          tunnel: w171 -> [w200]
          tunnel: [w200] -> w170
          tunnel: w152 -> [w199]
          tunnel: [w199] -> w151
          frame #0 {
            n946 = Wait (ms)(milliseconds to wait=u32 100) -> ()  [unwired: 1 out]
          }
        }
        n947 = call "IRSensorNIRead.vi"("error in (no error)"=w140, "Melexis_Cmmds"=w137, "Address"=u8 3, "device reference"=w151) -> ("error out"=w142:errorcluster, "Temperature"=w148:dbl, "device reference out"=w147:T6)  [unwired: 5 in]
        n948 = local write "error out"(w142) -> ()
        n949 = Unbundle By Name(w142) -> ("status"=w143:bool)
        n950 = case shown="False" w143 {
          tunnel: w167 -> [w185 _]
          tunnel: [w185 w186] -> w169
          frame False {
            n951 = local write "Temperature 3"(w185) -> ()
          }
          frame True {
            n952 = local read "Temperature 3"() -> (w186:dbl)
          }
        }
        n953 = call-poly <vilib>:"PID Control Input Filter.vi"("input"=w148) -> ("output"=w168:dbl)  [unwired: 4 in]
        n954 = flat-sequence {
          tunnel: w168 -> [w197]
          tunnel: [w197] -> w167
          tunnel: w147 -> [w196]
          tunnel: [w196] -> w145
          frame #0 {
            n955 = Wait (ms)(milliseconds to wait=u32 100) -> ()  [unwired: 1 out]
          }
        }
        n956 = call "IRSensorNIRead.vi"("error in (no error)"=w140, "Melexis_Cmmds"=w137, "Address"=u8 4, "device reference"=w145) -> ("error out"=w132:errorcluster, "Temperature"=w144:dbl, "device reference out"=w139:T6)  [unwired: 5 in]
        n957 = local write "error out"(w132) -> ()
        n958 = Unbundle By Name(w132) -> ("status"=w134:bool)
        n959 = case shown="True" w134 {
          tunnel: w165 -> [w183 _]
          tunnel: [w183 w184] -> w175
          frame False {
            n960 = local write "Temperature 4"(w183) -> ()
          }
          frame True {
            n961 = local read "Temperature 4"() -> (w184:dbl)
          }
        }
        n962 = call-poly <vilib>:"PID Control Input Filter.vi"("input"=w144) -> ("output"=w166:dbl)  [unwired: 4 in]
        n963 = flat-sequence {
          tunnel: w166 -> [w194]
          tunnel: [w194] -> w165
          tunnel: w139 -> [w193]
          tunnel: [w193] -> w138
          frame #0 {
            n964 = Wait (ms)(milliseconds to wait=u32 100) -> ()  [unwired: 1 out]
          }
        }
        n965 = call "IRSensorNIRead.vi"("error in (no error)"=w140, "Melexis_Cmmds"=w137, "Address"=u8 5, "device reference"=w138) -> ("error out"=w135:errorcluster, "Temperature"=w136:dbl)  [unwired: 5 in, 1 out]
        n966 = local write "error out"(w135) -> ()
        n967 = flat-sequence {
          tunnel: w164 -> [w191]
          tunnel: [w191] -> w163
          frame #0 {
            n968 = Wait (ms)(milliseconds to wait=u32 100) -> ()  [unwired: 1 out]
          }
        }
        n969 = Unbundle By Name(w135) -> ("status"=w133:bool)
        n970 = call-poly <vilib>:"PID Control Input Filter.vi"("input"=w136) -> ("output"=w164:dbl)  [unwired: 4 in]
        n971 = local write "error out"(w140) -> ()
        n972 = Build Array(w177, w176, w169, w175, w163) -> (w179:dbl[])
        n973 = Array To Cluster(array=w179) -> (cluster=→"Teperature Chart":T3)
        n974 = case shown="False" w133 {
          tunnel: w163 -> [w181 _]
          tunnel: [w181 w182] -> w174
          frame False {
            n975 = local write "Temperature 5"(w181) -> ()
          }
          frame True {
            n976 = local read "Temperature 5"() -> (w182:dbl)
          }
        }
        n977 = script code="MATLAB script"("T1"=w177, "T2"=w176, "T3"=w169, "T4"=w175, "T5"=w174) -> ()  [unwired: 1 in, 1 out]
      }
      n978 = while {
        stop <- w95 stop-if-true
        n979 = local read "Pump setpoint(ul/min) 1"() -> (w98:dbl)
        n980 = local read "Pump setpoint(ul/min) 2"() -> (w94:dbl)
        n981 = local read "Pump setpoint(ul/min) 3"() -> (w93:dbl)
        n982 = local read "Pump setpoint(ul/min) 4"() -> (w92:dbl)
        n983 = local read "Pump setpoint(ul/min) 5"() -> (w91:dbl)
        n984 = local read "Pump setpoint(ul/min) 6"() -> (w90:dbl)
        n985 = Build Array(w98, w94, w93, w92, w91, w90) -> (w99:dbl[])
        n986 = Array To Cluster(array=w99) -> (cluster=→"Pump Setpoints Chart":T3)
        n987 = Wait (ms)(milliseconds to wait=u32 5000) -> ()  [unwired: 1 out]
        n988 = local read "Stop"() -> (w95:bool)
      }
      n989 = while {
        stop <- w77 stop-if-true
        n990 = local read "System Error"() -> (w76:bool)
        n991 = Wait (ms)(milliseconds to wait=u32 300) -> ()  [unwired: 1 out]
        n992 = case shown="False" w76 {
          tunnel: [w81 w82] -> w74
          frame False {
            w78 = u16 2 items=["System  Error", "System Running", "System Standby"] ("System Status")
            w79 = u16 1 items=["System  Error", "System Running", "System Standby"] ("System Status")
            n993 = local read "running?"() -> (w80:bool)
            n994 = Select(t=w79, s=w80, f=w78) -> (s? t:f=w81:u16)
          }
          frame True {
            w82 = u16 0 items=["System  Error", "System Running", "System Standby"] ("System Status")
          }
        }
        n995 = local read "Stop"() -> (w77:bool)
        n996 = local write "System Status"(w74) -> ()
      }
      n997 = while {
        tunnel: w61 -> [w83]
        stop <- w89 stop-if-true
        n998 = call-poly <vilib>:"Analog Read.vi"("Analog Channel"=u8 0, "LINX Resource"=w83) -> ("Voltage"=w84:dbl)  [unwired: 6 in, 3 out]
        "Phase_Sensor_voltage" <- w84
        n999 = Wait (ms)(milliseconds to wait=u32 300) -> ()  [unwired: 1 out]
        n1000 = Build Array(w84) -> (w86:dbl[])
        n1001 = Array To Cluster(array=w86) -> (cluster=→"Phase Sensor Chart":T3)
        n1002 = local read "Stop"() -> (w89:bool)
      }
      n1003 = while {
        stop <- w71 stop-if-true
        n1004 = script code="TempArrLED=circshift(TempArrLED,9);\nTempArrLED(10)=T1;\navgTemp = mean(TempArrLED);"() -> ("avgTemp"=w67:dbl)  [unwired: 1 in, 1 out]
        n1005 = Wait (ms)(milliseconds to wait=u32 1000) -> ()  [unwired: 1 out]
        n1006 = Greater?(x=w67, y=110.0) -> (0:w69:bool)
        n1007 = case shown="True" w69 {
          frame False {
          }
          frame True {
            w73 = TRUE
            n1008 = local write "Stop"(w73) -> ()
            n1009 = local write "System Error"(w73) -> ()
            n1010 = local write "Error Message"("Temperature in Bay 2 is above 110'C") -> ()
            n1011 = script code="system_error = 1;"() -> ()  [unwired: 1 in, 1 out]
          }
        }
        n1012 = local read "Stop"() -> (w71:bool)
      }
      n1013 = while {
        tunnel: w61 -> [w102]
        stop <- w127 stop-if-true
        w109 = 270
        w103 = 600
        w104 = 600
        # "Read Pressure and Flowrate"
        n1014 = local read "Stop"() -> (w127:bool)
        n1015 = call-poly <vilib>:"Analog Read.vi"("AI Channel(s)"=i32[] [14, 15, 14, 15], "LINX Resource"=w102) -> ("Voltages"=w100:dbl[])  [unwired: 6 in, 3 out]
        n1016 = Index Array(array=w100, index=1) -> (element=w123:dbl)
        n1017 = Index Array(array=w100, index=0) -> (element=w124:dbl)
        n1018 = call-poly <vilib>:"PID Control Input Filter.vi"("input"=w123) -> ("output"=w116:dbl)  [unwired: 4 in]
        n1019 = call-poly <vilib>:"PID Control Input Filter.vi"("input"=w124) -> ("output"=w115:dbl)  [unwired: 4 in]
        n1020 = Multiply(x=104.96 ("y"), y=w116) -> (x*y=w117:dbl)
        n1021 = Multiply(x=104.96 ("y"), y=w115) -> (x*y=w120:dbl)
        n1022 = Subtract(x=w117, y=24.077) -> (x-y=w107:dbl)
        n1023 = Subtract(x=w120, y=24.077) -> (x-y=w108:dbl)
        n1024 = Build Array(w104, w103) -> (w112:i32[])
        n1025 = Array To Cluster(array=w112) -> (cluster=→"Flowrate Chart":T4)
        n1026 = Build Array(w108, w107) -> (w113:dbl[])
        n1027 = local write "Flowrate Sensor 1"(w104) -> ()
        n1028 = local write "Flowrate Sensor 2"(w103) -> ()
        n1029 = local write "Pressure 1"(w108) -> ()
        n1030 = local write "Pressure 2"(w107) -> ()
        n1031 = Array To Cluster(array=w113) -> (cluster=→"Pressure Chart":T3)
        n1032 = Wait (ms)(milliseconds to wait=u32 500) -> ()  [unwired: 1 out]
        n1033 = script code="MATLAB script"("F1"=w104, "F2"=w103, "Pres1"=w108, "Pres2"=w107) -> ()  [unwired: 1 in, 1 out]
        n1034 = Greater?(x=w107, y=w109) -> (0:w105:bool)
        n1035 = Greater?(x=w108, y=w109) -> (0:w106:bool)
        n1036 = case shown="False" w106 {
          frame False {
          }
          frame True {
            w131 = TRUE ("Stop")
            n1037 = local write "System Error"(w131) -> ()
            n1038 = local write "Stop"(w131) -> ()
            n1039 = local write "Error Message"("Pressure Sensor 1 readings above 250psi") -> ()
            n1040 = script code="system_error = 1;"() -> ()  [unwired: 1 in, 1 out]
          }
        }
        n1041 = case shown="True" w105 {
          frame False {
          }
          frame True {
            w129 = TRUE ("Stop")
            n1042 = local write "System Error"(w129) -> ()
            n1043 = local write "Error Message"("Pressure Sensor 2 readings above 250psi") -> ()
            n1044 = local write "Stop"(w129) -> ()
            n1045 = script code="system_error = 1;"() -> ()  [unwired: 1 in, 1 out]
          }
        }
      }
    }
    frame #3 {
      # "Save and close xml and excel file"
      n1046 = script code="if exist('xl_file','var') & exist('xlApp','var')\n  xlWorkbook.SaveAs(xl_file);\n  xlWorkbook.Close;\n  xlApp.Quit;\n  xlApp.delete;\nend"() -> ()  [unwired: 1 in, 1 out]
    }
    frame #4 {
      w1414 = string[] ["e", "f", "g", "h", "i", "j"]
      # "End communication to hardware"
      n1047 = local read "Syringe_pump?"() -> (w1412:bool)
      n1048 = local read "COMM Port:: Harvard Syringe Pump"() -> (w1413:refnum<visa-resource-name>)
      n1049 = local read "IR Sensor Device"() -> (w1411:T6)
      n1050 = local read "COMM Port :: Milligat Pumps"() -> (w1416:refnum<visa-resource-name>)
      n1051 = call <vilib>:"Close.vi"("LINX Resource"=w1410) -> ()  [unwired: 10 in, 1 out]
      n1052 = Array Size(array=w1414) -> (size(s)=w1415:i32)
      n1053 = case shown="True" w1412 {
        tunnel: w1413 -> [_ w1417]
        frame False {
        }
        frame True {
          n1054 = call <instrlib>:"Stop Pump.vi"("VISA resource name"=w1417) -> ()  [unwired: 9 in, 2 out]
        }
      }
      n1055 = for {
        N: w1415 -> [_]
        tunnel: w1414 -> [w1418] mode=indexing
        tunnel: w1416 -> [w1419]
        n1056 = call "PumpStop.vi"("Pump Address"=w1418, "Pump COMM Port"=w1419) -> ()  [unwired: 9 in, 1 out]
        n1057 = Wait (ms)(milliseconds to wait=u32 300) -> ()  [unwired: 1 out]
      }
      n1058 = call-poly <vilib>:"NI-845x Close Reference.vi"("device reference"=w1411) -> ()  [unwired: 10 in, 1 out]
    }
    frame #5 {
      # "Display Error Messages if necessary"
      n1059 = local read "Error Message"() -> (w1421:string)
      n1060 = One Button Dialog(message=w1421) -> ()  [unwired: 1 in, 1 out]
    }
  }
